vi "Calibrate Sensor.vi"(0 "Sensor":T4={"Sensor Name"="AI 0", "Sensor Info"={"Manufacturer"="", "Model"="", "Serial Number"=""}, "Last Cal Info"={"Last Calibration Date"=3153138208.25, "Calibrator"="", "Cal Duration"=0}, "Voltage Range"={"High Limit"=0.0, "Low Limit"=10.0}, "EGU Range"={"High Limit"=0.0, "Low Limit"=10.0}, "Units"="Volts", "Calibration Type"=enum."Calibrate Analog", "EGU List"=[0.0, 10000.0], "Voltage List"=[0.0, 5.0], "Coefficients"=[3.658184866139891e-14, 1999.9999999999998], "Order"=1, "Algorithm"=enum."SVD", "Max Error % of Full Scale"=0.0, "Max Mean Squared Error"=0.0, "Use Error %"=FALSE, "Use MSE"=FALSE, "Allow Manual Entry"=FALSE, "Max Stability Error"=2.0, "Max Error % of Reading"=0.0, "Use Error % of Reading"=FALSE}, 1 "System Ref":tag, 2 "TCP Stream Ref":refnum<vi>, 5 "Channel Info":T5={"Channel"="0-10V AI #0", "Description"="0-10V AI #0", "Acquire"=FALSE, "Sensor"="AI 0", "Chg Sensor"=FALSE, "Cal Date"="", "Offset"=0.0, "Span"=0.0, "Cal"=FALSE, "Test Limits"=FALSE, "Type"="", "Data Index"=0}, 7 "Cal Base Path":path, 9 "System Type":T1, 11 "Devices":T2=[{"Device"=2, "Channels"=[{"Channel ID"="OB0!SC1!MD2!0", "Channel Name"="0-10V AI #0 TRDC.1", "Channel Type"=enum."Voltage", "Selected Sensor"="WTI func gen", "Alarm Config"={"Action"=enum."Disabled", "Low Limit"=0.0, "High Limit"=0.0}, "Thermocouple Info"={"Thermocouple Type"=0, "Temperature Units"=0, "Temperature Low Limit"=0.0, "Temperature High Limit"=0.0, "CJC Sensor Type"=0, "Thermistor Excitation"=0, "CJC Channel ID"=0, "Dedicated CJTEMP for Channel"=0, "Use CALGND"=0, "Dedicated CALGND for Channel"=0}}, {"Channel ID"="OB0!SC1!MD1!0", "Channel Name"="J-TYPE TC #0", "Channel Type"=enum."Thermocouple", "Selected Sensor"="Hardware", "Alarm Config"={"Action"=enum."Disabled", "Low Limit"=0.0, "High Limit"=0.0}, "Thermocouple Info"={"Thermocouple Type"=2, "Temperature Units"=0, "Temperature Low Limit"=-60.0, "Temperature High Limit"=200.0, "CJC Sensor Type"=1, "Thermistor Excitation"=0, "CJC Channel ID"=0, "Dedicated CJTEMP for Channel"=0, "Use CALGND"=0, "Dedicated CALGND for Channel"=0}}, {"Channel ID"="OB0!SC1!MD1!1", "Channel Name"="J-TYPE TC #1", "Channel Type"=enum."Thermocouple", "Selected Sensor"="Hardware", "Alarm Config"={"Action"=enum."Disabled", "Low Limit"=0.0, "High Limit"=0.0}, "Thermocouple Info"={"Thermocouple Type"=2, "Temperature Units"=0, "Temperature Low Limit"=-60.0, "Temperature High Limit"=200.0, "CJC Sensor Type"=1, "Thermistor Excitation"=0, "CJC Channel ID"=0, "Dedicated CJTEMP for Channel"=0, "Use CALGND"=0, "Dedicated CALGND for Channel"=0}}, {"Channel ID"="OB0!SC1!MD1!2", "Channel Name"="J-TYPE TC #2", "Channel Type"=enum."Thermocouple", "Selected Sensor"="Hardware", "Alarm Config"={"Action"=enum."Disabled", "Low Limit"=0.0, "High Limit"=0.0}, "Thermocouple Info"={"Thermocouple Type"=2, "Temperature Units"=0, "Temperature Low Limit"=-60.0, "Temperature High Limit"=200.0, "CJC Sensor Type"=1, "Thermistor Excitation"=0, "CJC Channel ID"=0, "Dedicated CJTEMP for Channel"=0, "Use CALGND"=0, "Dedicated CALGND for Channel"=0}}, {"Channel ID"="OB0!SC1!MD1!3", "Channel Name"="J-TYPE TC #3", "Channel Type"=enum."Thermocouple", "Selected Sensor"="Hardware", "Alarm Config"={"Action"=enum."Disabled", "Low Limit"=0.0, "High Limit"=0.0}, "Thermocouple Info"={"Thermocouple Type"=2, "Temperature Units"=0, "Temperature Low Limit"=-60.0, "Temperature High Limit"=200.0, "CJC Sensor Type"=1, "Thermistor Excitation"=0, "CJC Channel ID"=0, "Dedicated CJTEMP for Channel"=0, "Use CALGND"=0, "Dedicated CALGND for Channel"=0}}, {"Channel ID"="OB0!SC1!MD1!4", "Channel Name"="J-TYPE TC #4", "Channel Type"=enum."Thermocouple", "Selected Sensor"="Hardware", "Alarm Config"={"Action"=enum."Disabled", "Low Limit"=0.0, "High Limit"=0.0}, "Thermocouple Info"={"Thermocouple Type"=2, "Temperature Units"=0, "Temperature Low Limit"=-60.0, "Temperature High Limit"=200.0, "CJC Sensor Type"=1, "Thermistor Excitation"=0, "CJC Channel ID"=0, "Dedicated CJTEMP for Channel"=0, "Use CALGND"=0, "Dedicated CALGND for Channel"=0}}, {"Channel ID"="OB0!SC1!MD1!5", "Channel Name"="J-TYPE TC #5", "Channel Type"=enum."Thermocouple", "Selected Sensor"="Hardware", "Alarm Config"={"Action"=enum."Disabled", "Low Limit"=0.0, "High Limit"=0.0}, "Thermocouple Info"={"Thermocouple Type"=2, "Temperature Units"=0, "Temperature Low Limit"=-60.0, "Temperature High Limit"=200.0, "CJC Sensor Type"=1, "Thermistor Excitation"=0, "CJC Channel ID"=0, "Dedicated CJTEMP for Channel"=0, "Use CALGND"=0, "Dedicated CALGND for Channel"=0}}, {"Channel ID"="OB0!SC1!MD1!6", "Channel Name"="J-TYPE TC #6", "Channel Type"=enum."Thermocouple", "Selected Sensor"="Hardware", "Alarm Config"={"Action"=enum."Disabled", "Low Limit"=0.0, "High Limit"=0.0}, "Thermocouple Info"={"Thermocouple Type"=2, "Temperature Units"=0, "Temperature Low Limit"=-60.0, "Temperature High Limit"=200.0, "CJC Sensor Type"=1, "Thermistor Excitation"=0, "CJC Channel ID"=0, "Dedicated CJTEMP for Channel"=0, "Use CALGND"=0, "Dedicated CALGND for Channel"=0}}, {"Channel ID"="OB0!SC1!MD1!7", "Channel Name"="J-TYPE TC #7", "Channel Type"=enum."Thermocouple", "Selected Sensor"="Hardware", "Alarm Config"={"Action"=enum."Disabled", "Low Limit"=0.0, "High Limit"=0.0}, "Thermocouple Info"={"Thermocouple Type"=2, "Temperature Units"=0, "Temperature Low Limit"=-60.0, "Temperature High Limit"=200.0, "CJC Sensor Type"=1, "Thermistor Excitation"=0, "CJC Channel ID"=0, "Dedicated CJTEMP for Channel"=0, "Use CALGND"=0, "Dedicated CALGND for Channel"=0}}, {"Channel ID"="OB0!SC1!MD1!8", "Channel Name"="J-TYPE TC #8", "Channel Type"=enum."Thermocouple", "Selected Sensor"="Hardware", "Alarm Config"={"Action"=enum."Disabled", "Low Limit"=0.0, "High Limit"=0.0}, "Thermocouple Info"={"Thermocouple Type"=2, "Temperature Units"=0, "Temperature Low Limit"=-60.0, "Temperature High Limit"=200.0, "CJC Sensor Type"=1, "Thermistor Excitation"=0, "CJC Channel ID"=0, "Dedicated CJTEMP for Channel"=0, "Use CALGND"=0, "Dedicated CALGND for Channel"=0}}, {"Channel ID"="OB0!SC1!MD1!9", "Channel Name"="J-TYPE TC #9", "Channel Type"=enum."Thermocouple", "Selected Sensor"="Hardware", "Alarm Config"={"Action"=enum."Disabled", "Low Limit"=0.0, "High Limit"=0.0}, "Thermocouple Info"={"Thermocouple Type"=2, "Temperature Units"=0, "Temperature Low Limit"=-60.0, "Temperature High Limit"=200.0, "CJC Sensor Type"=1, "Thermistor Excitation"=0, "CJC Channel ID"=0, "Dedicated CJTEMP for Channel"=0, "Use CALGND"=0, "Dedicated CALGND for Channel"=0}}, {"Channel ID"="OB0!SC1!MD1!10", "Channel Name"="J-TYPE TC #10", "Channel Type"=enum."Thermocouple", "Selected Sensor"="Hardware", "Alarm Config"={"Action"=enum."Disabled", "Low Limit"=0.0, "High Limit"=0.0}, "Thermocouple Info"={"Thermocouple Type"=2, "Temperature Units"=0, "Temperature Low Limit"=-60.0, "Temperature High Limit"=200.0, "CJC Sensor Type"=1, "Thermistor Excitation"=0, "CJC Channel ID"=0, "Dedicated CJTEMP for Channel"=0, "Use CALGND"=0, "Dedicated CALGND for Channel"=0}}, {"Channel ID"="OB0!SC1!MD1!11", "Channel Name"="J-TYPE TC #11", "Channel Type"=enum."Thermocouple", "Selected Sensor"="Hardware", "Alarm Config"={"Action"=enum."Disabled", "Low Limit"=0.0, "High Limit"=0.0}, "Thermocouple Info"={"Thermocouple Type"=2, "Temperature Units"=0, "Temperature Low Limit"=-60.0, "Temperature High Limit"=200.0, "CJC Sensor Type"=1, "Thermistor Excitation"=0, "CJC Channel ID"=0, "Dedicated CJTEMP for Channel"=0, "Use CALGND"=0, "Dedicated CALGND for Channel"=0}}, {"Channel ID"="OB0!SC1!MD1!12", "Channel Name"="J-TYPE TC #12", "Channel Type"=enum."Thermocouple", "Selected Sensor"="Hardware", "Alarm Config"={"Action"=enum."Disabled", "Low Limit"=0.0, "High Limit"=0.0}, "Thermocouple Info"={"Thermocouple Type"=2, "Temperature Units"=0, "Temperature Low Limit"=-60.0, "Temperature High Limit"=200.0, "CJC Sensor Type"=1, "Thermistor Excitation"=0, "CJC Channel ID"=0, "Dedicated CJTEMP for Channel"=0, "Use CALGND"=0, "Dedicated CALGND for Channel"=0}}, {"Channel ID"="OB0!SC1!MD1!13", "Channel Name"="J-TYPE TC #13", "Channel Type"=enum."Thermocouple", "Selected Sensor"="Hardware", "Alarm Config"={"Action"=enum."Disabled", "Low Limit"=0.0, "High Limit"=0.0}, "Thermocouple Info"={"Thermocouple Type"=2, "Temperature Units"=0, "Temperature Low Limit"=-60.0, "Temperature High Limit"=200.0, "CJC Sensor Type"=1, "Thermistor Excitation"=0, "CJC Channel ID"=0, "Dedicated CJTEMP for Channel"=0, "Use CALGND"=0, "Dedicated CALGND for Channel"=0}}, {"Channel ID"="OB0!SC1!MD1!14", "Channel Name"="J-TYPE TC #14", "Channel Type"=enum."Thermocouple", "Selected Sensor"="Hardware", "Alarm Config"={"Action"=enum."Disabled", "Low Limit"=0.0, "High Limit"=0.0}, "Thermocouple Info"={"Thermocouple Type"=2, "Temperature Units"=0, "Temperature Low Limit"=-60.0, "Temperature High Limit"=200.0, "CJC Sensor Type"=1, "Thermistor Excitation"=0, "CJC Channel ID"=0, "Dedicated CJTEMP for Channel"=0, "Use CALGND"=0, "Dedicated CALGND for Channel"=0}}, {"Channel ID"="OB0!SC1!MD1!15", "Channel Name"="J-TYPE TC #15", "Channel Type"=enum."Thermocouple", "Selected Sensor"="Hardware", "Alarm Config"={"Action"=enum."Disabled", "Low Limit"=0.0, "High Limit"=0.0}, "Thermocouple Info"={"Thermocouple Type"=2, "Temperature Units"=0, "Temperature Low Limit"=-60.0, "Temperature High Limit"=200.0, "CJC Sensor Type"=1, "Thermistor Excitation"=0, "CJC Channel ID"=0, "Dedicated CJTEMP for Channel"=0, "Use CALGND"=0, "Dedicated CALGND for Channel"=0}}, {"Channel ID"="OB0!SC1!MD1!16", "Channel Name"="T-TYPE TC #16", "Channel Type"=enum."Thermocouple", "Selected Sensor"="Hardware", "Alarm Config"={"Action"=enum."Disabled", "Low Limit"=0.0, "High Limit"=0.0}, "Thermocouple Info"={"Thermocouple Type"=6, "Temperature Units"=0, "Temperature Low Limit"=-60.0, "Temperature High Limit"=200.0, "CJC Sensor Type"=1, "Thermistor Excitation"=0, "CJC Channel ID"=0, "Dedicated CJTEMP for Channel"=0, "Use CALGND"=0, "Dedicated CALGND for Channel"=0}}, {"Channel ID"="OB0!SC1!MD1!17", "Channel Name"="T-TYPE TC #17", "Channel Type"=enum."Thermocouple", "Selected Sensor"="Hardware", "Alarm Config"={"Action"=enum."Disabled", "Low Limit"=0.0, "High Limit"=0.0}, "Thermocouple Info"={"Thermocouple Type"=6, "Temperature Units"=0, "Temperature Low Limit"=-60.0, "Temperature High Limit"=200.0, "CJC Sensor Type"=1, "Thermistor Excitation"=0, "CJC Channel ID"=0, "Dedicated CJTEMP for Channel"=0, "Use CALGND"=0, "Dedicated CALGND for Channel"=0}}, {"Channel ID"="OB0!SC1!MD1!18", "Channel Name"="T-TYPE TC #18", "Channel Type"=enum."Thermocouple", "Selected Sensor"="Hardware", "Alarm Config"={"Action"=enum."Disabled", "Low Limit"=0.0, "High Limit"=0.0}, "Thermocouple Info"={"Thermocouple Type"=6, "Temperature Units"=0, "Temperature Low Limit"=-60.0, "Temperature High Limit"=200.0, "CJC Sensor Type"=1, "Thermistor Excitation"=0, "CJC Channel ID"=0, "Dedicated CJTEMP for Channel"=0, "Use CALGND"=0, "Dedicated CALGND for Channel"=0}}, {"Channel ID"="OB0!SC1!MD1!19", "Channel Name"="T-TYPE TC #19", "Channel Type"=enum."Thermocouple", "Selected Sensor"="Hardware", "Alarm Config"={"Action"=enum."Disabled", "Low Limit"=0.0, "High Limit"=0.0}, "Thermocouple Info"={"Thermocouple Type"=6, "Temperature Units"=0, "Temperature Low Limit"=-60.0, "Temperature High Limit"=200.0, "CJC Sensor Type"=1, "Thermistor Excitation"=0, "CJC Channel ID"=0, "Dedicated CJTEMP for Channel"=0, "Use CALGND"=0, "Dedicated CALGND for Channel"=0}}, {"Channel ID"="OB0!SC1!MD1!20", "Channel Name"="T-TYPE TC #20", "Channel Type"=enum."Thermocouple", "Selected Sensor"="Hardware", "Alarm Config"={"Action"=enum."Disabled", "Low Limit"=0.0, "High Limit"=0.0}, "Thermocouple Info"={"Thermocouple Type"=6, "Temperature Units"=0, "Temperature Low Limit"=-60.0, "Temperature High Limit"=200.0, "CJC Sensor Type"=1, "Thermistor Excitation"=0, "CJC Channel ID"=0, "Dedicated CJTEMP for Channel"=0, "Use CALGND"=0, "Dedicated CALGND for Channel"=0}}, {"Channel ID"="OB0!SC1!MD1!21", "Channel Name"="T-TYPE TC #21", "Channel Type"=enum."Thermocouple", "Selected Sensor"="Hardware", "Alarm Config"={"Action"=enum."Disabled", "Low Limit"=0.0, "High Limit"=0.0}, "Thermocouple Info"={"Thermocouple Type"=6, "Temperature Units"=0, "Temperature Low Limit"=-60.0, "Temperature High Limit"=200.0, "CJC Sensor Type"=1, "Thermistor Excitation"=0, "CJC Channel ID"=0, "Dedicated CJTEMP for Channel"=0, "Use CALGND"=0, "Dedicated CALGND for Channel"=0}}, {"Channel ID"="OB0!SC1!MD1!22", "Channel Name"="T-TYPE TC #22", "Channel Type"=enum."Thermocouple", "Selected Sensor"="Hardware", "Alarm Config"={"Action"=enum."Disabled", "Low Limit"=0.0, "High Limit"=0.0}, "Thermocouple Info"={"Thermocouple Type"=6, "Temperature Units"=0, "Temperature Low Limit"=-60.0, "Temperature High Limit"=200.0, "CJC Sensor Type"=1, "Thermistor Excitation"=0, "CJC Channel ID"=0, "Dedicated CJTEMP for Channel"=0, "Use CALGND"=0, "Dedicated CALGND for Channel"=0}}, {"Channel ID"="OB0!SC1!MD1!23", "Channel Name"="T-TYPE TC #23", "Channel Type"=enum."Thermocouple", "Selected Sensor"="Hardware", "Alarm Config"={"Action"=enum."Disabled", "Low Limit"=0.0, "High Limit"=0.0}, "Thermocouple Info"={"Thermocouple Type"=6, "Temperature Units"=0, "Temperature Low Limit"=-60.0, "Temperature High Limit"=200.0, "CJC Sensor Type"=1, "Thermistor Excitation"=0, "CJC Channel ID"=0, "Dedicated CJTEMP for Channel"=0, "Use CALGND"=0, "Dedicated CALGND for Channel"=0}}, {"Channel ID"="OB0!SC1!MD1!24", "Channel Name"="T-TYPE TC #24", "Channel Type"=enum."Thermocouple", "Selected Sensor"="Hardware", "Alarm Config"={"Action"=enum."Disabled", "Low Limit"=0.0, "High Limit"=0.0}, "Thermocouple Info"={"Thermocouple Type"=6, "Temperature Units"=0, "Temperature Low Limit"=-60.0, "Temperature High Limit"=200.0, "CJC Sensor Type"=1, "Thermistor Excitation"=0, "CJC Channel ID"=0, "Dedicated CJTEMP for Channel"=0, "Use CALGND"=0, "Dedicated CALGND for Channel"=0}}, {"Channel ID"="OB0!SC1!MD1!25", "Channel Name"="T-TYPE TC #25", "Channel Type"=enum."Thermocouple", "Selected Sensor"="Hardware", "Alarm Config"={"Action"=enum."Disabled", "Low Limit"=0.0, "High Limit"=0.0}, "Thermocouple Info"={"Thermocouple Type"=6, "Temperature Units"=0, "Temperature Low Limit"=-60.0, "Temperature High Limit"=200.0, "CJC Sensor Type"=1, "Thermistor Excitation"=0, "CJC Channel ID"=0, "Dedicated CJTEMP for Channel"=0, "Use CALGND"=0, "Dedicated CALGND for Channel"=0}}, {"Channel ID"="OB0!SC1!MD1!26", "Channel Name"="T-TYPE TC #26", "Channel Type"=enum."Thermocouple", "Selected Sensor"="Hardware", "Alarm Config"={"Action"=enum."Disabled", "Low Limit"=0.0, "High Limit"=0.0}, "Thermocouple Info"={"Thermocouple Type"=6, "Temperature Units"=0, "Temperature Low Limit"=-60.0, "Temperature High Limit"=200.0, "CJC Sensor Type"=1, "Thermistor Excitation"=0, "CJC Channel ID"=0, "Dedicated CJTEMP for Channel"=0, "Use CALGND"=0, "Dedicated CALGND for Channel"=0}}, {"Channel ID"="OB0!SC1!MD1!27", "Channel Name"="T-TYPE TC #27", "Channel Type"=enum."Thermocouple", "Selected Sensor"="Hardware", "Alarm Config"={"Action"=enum."Disabled", "Low Limit"=0.0, "High Limit"=0.0}, "Thermocouple Info"={"Thermocouple Type"=6, "Temperature Units"=0, "Temperature Low Limit"=-60.0, "Temperature High Limit"=200.0, "CJC Sensor Type"=1, "Thermistor Excitation"=0, "CJC Channel ID"=0, "Dedicated CJTEMP for Channel"=0, "Use CALGND"=0, "Dedicated CALGND for Channel"=0}}, {"Channel ID"="OB0!SC1!MD1!28", "Channel Name"="T-TYPE TC #28", "Channel Type"=enum."Thermocouple", "Selected Sensor"="Hardware", "Alarm Config"={"Action"=enum."Disabled", "Low Limit"=0.0, "High Limit"=0.0}, "Thermocouple Info"={"Thermocouple Type"=6, "Temperature Units"=0, "Temperature Low Limit"=-60.0, "Temperature High Limit"=200.0, "CJC Sensor Type"=1, "Thermistor Excitation"=0, "CJC Channel ID"=0, "Dedicated CJTEMP for Channel"=0, "Use CALGND"=0, "Dedicated CALGND for Channel"=0}}, {"Channel ID"="OB0!SC1!MD1!29", "Channel Name"="T-TYPE TC #29", "Channel Type"=enum."Thermocouple", "Selected Sensor"="Hardware", "Alarm Config"={"Action"=enum."Disabled", "Low Limit"=0.0, "High Limit"=0.0}, "Thermocouple Info"={"Thermocouple Type"=6, "Temperature Units"=0, "Temperature Low Limit"=-60.0, "Temperature High Limit"=200.0, "CJC Sensor Type"=1, "Thermistor Excitation"=0, "CJC Channel ID"=0, "Dedicated CJTEMP for Channel"=0, "Use CALGND"=0, "Dedicated CALGND for Channel"=0}}, {"Channel ID"="OB0!SC1!MD1!30", "Channel Name"="T-TYPE TC #30", "Channel Type"=enum."Thermocouple", "Selected Sensor"="Hardware", "Alarm Config"={"Action"=enum."Disabled", "Low Limit"=0.0, "High Limit"=0.0}, "Thermocouple Info"={"Thermocouple Type"=6, "Temperature Units"=0, "Temperature Low Limit"=-60.0, "Temperature High Limit"=200.0, "CJC Sensor Type"=1, "Thermistor Excitation"=0, "CJC Channel ID"=0, "Dedicated CJTEMP for Channel"=0, "Use CALGND"=0, "Dedicated CALGND for Channel"=0}}, {"Channel ID"="OB0!SC1!MD1!31", "Channel Name"="T-TYPE TC #31", "Channel Type"=enum."Thermocouple", "Selected Sensor"="Hardware", "Alarm Config"={"Action"=enum."Disabled", "Low Limit"=0.0, "High Limit"=0.0}, "Thermocouple Info"={"Thermocouple Type"=6, "Temperature Units"=0, "Temperature Low Limit"=-60.0, "Temperature High Limit"=200.0, "CJC Sensor Type"=1, "Thermistor Excitation"=0, "CJC Channel ID"=0, "Dedicated CJTEMP for Channel"=0, "Use CALGND"=0, "Dedicated CALGND for Channel"=0}}, {"Channel ID"="OB0!SC1!MD2!0", "Channel Name"="0-10V AI #0 TRDC.1", "Channel Type"=enum."Voltage", "Selected Sensor"="WTI func gen", "Alarm Config"={"Action"=enum."Disabled", "Low Limit"=0.0, "High Limit"=0.0}, "Thermocouple Info"={"Thermocouple Type"=0, "Temperature Units"=0, "Temperature Low Limit"=-60.0, "Temperature High Limit"=200.0, "CJC Sensor Type"=1, "Thermistor Excitation"=0, "CJC Channel ID"=0, "Dedicated CJTEMP for Channel"=0, "Use CALGND"=0, "Dedicated CALGND for Channel"=0}}, {"Channel ID"="OB0!SC1!MD2!1", "Channel Name"="0-10V AI #1 TRDC.2", "Channel Type"=enum."Voltage", "Selected Sensor"="WTI func gen", "Alarm Config"={"Action"=enum."Disabled", "Low Limit"=0.0, "High Limit"=0.0}, "Thermocouple Info"={"Thermocouple Type"=0, "Temperature Units"=0, "Temperature Low Limit"=-60.0, "Temperature High Limit"=200.0, "CJC Sensor Type"=1, "Thermistor Excitation"=0, "CJC Channel ID"=0, "Dedicated CJTEMP for Channel"=0, "Use CALGND"=0, "Dedicated CALGND for Channel"=0}}, {"Channel ID"="OB0!SC1!MD2!2", "Channel Name"="0-10V AI #2 TRDC.3", "Channel Type"=enum."Voltage", "Selected Sensor"="WTI func gen", "Alarm Config"={"Action"=enum."Disabled", "Low Limit"=0.0, "High Limit"=0.0}, "Thermocouple Info"={"Thermocouple Type"=0, "Temperature Units"=0, "Temperature Low Limit"=-60.0, "Temperature High Limit"=200.0, "CJC Sensor Type"=1, "Thermistor Excitation"=0, "CJC Channel ID"=0, "Dedicated CJTEMP for Channel"=0, "Use CALGND"=0, "Dedicated CALGND for Channel"=0}}, {"Channel ID"="OB0!SC1!MD2!3", "Channel Name"="0-10V AI #3 TRDC.4", "Channel Type"=enum."Voltage", "Selected Sensor"="WTI func gen", "Alarm Config"={"Action"=enum."Disabled", "Low Limit"=0.0, "High Limit"=0.0}, "Thermocouple Info"={"Thermocouple Type"=0, "Temperature Units"=0, "Temperature Low Limit"=-60.0, "Temperature High Limit"=200.0, "CJC Sensor Type"=1, "Thermistor Excitation"=0, "CJC Channel ID"=0, "Dedicated CJTEMP for Channel"=0, "Use CALGND"=0, "Dedicated CALGND for Channel"=0}}, {"Channel ID"="OB0!SC1!MD2!4", "Channel Name"="0-10V AI #4 TRDC.5", "Channel Type"=enum."Voltage", "Selected Sensor"="WTI func gen", "Alarm Config"={"Action"=enum."Disabled", "Low Limit"=0.0, "High Limit"=0.0}, "Thermocouple Info"={"Thermocouple Type"=0, "Temperature Units"=0, "Temperature Low Limit"=-60.0, "Temperature High Limit"=200.0, "CJC Sensor Type"=1, "Thermistor Excitation"=0, "CJC Channel ID"=0, "Dedicated CJTEMP for Channel"=0, "Use CALGND"=0, "Dedicated CALGND for Channel"=0}}, {"Channel ID"="OB0!SC1!MD2!5", "Channel Name"="0-10V AI #5 TRDC.6", "Channel Type"=enum."Voltage", "Selected Sensor"="WTI func gen", "Alarm Config"={"Action"=enum."Disabled", "Low Limit"=0.0, "High Limit"=0.0}, "Thermocouple Info"={"Thermocouple Type"=0, "Temperature Units"=0, "Temperature Low Limit"=-60.0, "Temperature High Limit"=200.0, "CJC Sensor Type"=1, "Thermistor Excitation"=0, "CJC Channel ID"=0, "Dedicated CJTEMP for Channel"=0, "Use CALGND"=0, "Dedicated CALGND for Channel"=0}}, {"Channel ID"="OB0!SC1!MD2!6", "Channel Name"="0-10V AI #6 TRDC.7", "Channel Type"=enum."Voltage", "Selected Sensor"="WTI func gen", "Alarm Config"={"Action"=enum."Disabled", "Low Limit"=0.0, "High Limit"=0.0}, "Thermocouple Info"={"Thermocouple Type"=0, "Temperature Units"=0, "Temperature Low Limit"=-60.0, "Temperature High Limit"=200.0, "CJC Sensor Type"=1, "Thermistor Excitation"=0, "CJC Channel ID"=0, "Dedicated CJTEMP for Channel"=0, "Use CALGND"=0, "Dedicated CALGND for Channel"=0}}, {"Channel ID"="OB0!SC1!MD2!7", "Channel Name"="0-10V AI #7 TRDC.8", "Channel Type"=enum."Voltage", "Selected Sensor"="WTI func gen", "Alarm Config"={"Action"=enum."Disabled", "Low Limit"=0.0, "High Limit"=0.0}, "Thermocouple Info"={"Thermocouple Type"=0, "Temperature Units"=0, "Temperature Low Limit"=-60.0, "Temperature High Limit"=200.0, "CJC Sensor Type"=1, "Thermistor Excitation"=0, "CJC Channel ID"=0, "Dedicated CJTEMP for Channel"=0, "Use CALGND"=0, "Dedicated CALGND for Channel"=0}}, {"Channel ID"="OB0!SC1!MD2!8", "Channel Name"="0-10V AI #8 TRDC.9", "Channel Type"=enum."Voltage", "Selected Sensor"="WTI func gen", "Alarm Config"={"Action"=enum."Disabled", "Low Limit"=0.0, "High Limit"=0.0}, "Thermocouple Info"={"Thermocouple Type"=0, "Temperature Units"=0, "Temperature Low Limit"=-60.0, "Temperature High Limit"=200.0, "CJC Sensor Type"=1, "Thermistor Excitation"=0, "CJC Channel ID"=0, "Dedicated CJTEMP for Channel"=0, "Use CALGND"=0, "Dedicated CALGND for Channel"=0}}, {"Channel ID"="OB0!SC1!MD2!9", "Channel Name"="0-10V AI #9 TRDC.10", "Channel Type"=enum."Voltage", "Selected Sensor"="WTI func gen", "Alarm Config"={"Action"=enum."Disabled", "Low Limit"=0.0, "High Limit"=0.0}, "Thermocouple Info"={"Thermocouple Type"=0, "Temperature Units"=0, "Temperature Low Limit"=-60.0, "Temperature High Limit"=200.0, "CJC Sensor Type"=1, "Thermistor Excitation"=0, "CJC Channel ID"=0, "Dedicated CJTEMP for Channel"=0, "Use CALGND"=0, "Dedicated CALGND for Channel"=0}}, {"Channel ID"="OB0!SC1!MD2!10", "Channel Name"="0-10V AI #10 TRDC.11", "Channel Type"=enum."Voltage", "Selected Sensor"="WTI func gen", "Alarm Config"={"Action"=enum."Disabled", "Low Limit"=0.0, "High Limit"=0.0}, "Thermocouple Info"={"Thermocouple Type"=0, "Temperature Units"=0, "Temperature Low Limit"=-60.0, "Temperature High Limit"=200.0, "CJC Sensor Type"=1, "Thermistor Excitation"=0, "CJC Channel ID"=0, "Dedicated CJTEMP for Channel"=0, "Use CALGND"=0, "Dedicated CALGND for Channel"=0}}, {"Channel ID"="OB0!SC1!MD2!11", "Channel Name"="0-10V AI #11 TRDC.12", "Channel Type"=enum."Voltage", "Selected Sensor"="WTI func gen", "Alarm Config"={"Action"=enum."Disabled", "Low Limit"=0.0, "High Limit"=0.0}, "Thermocouple Info"={"Thermocouple Type"=0, "Temperature Units"=0, "Temperature Low Limit"=-60.0, "Temperature High Limit"=200.0, "CJC Sensor Type"=1, "Thermistor Excitation"=0, "CJC Channel ID"=0, "Dedicated CJTEMP for Channel"=0, "Use CALGND"=0, "Dedicated CALGND for Channel"=0}}, {"Channel ID"="OB0!SC1!MD2!12", "Channel Name"="0-10V AI #12 TRDC.13", "Channel Type"=enum."Voltage", "Selected Sensor"="WTI func gen", "Alarm Config"={"Action"=enum."Disabled", "Low Limit"=0.0, "High Limit"=0.0}, "Thermocouple Info"={"Thermocouple Type"=0, "Temperature Units"=0, "Temperature Low Limit"=-60.0, "Temperature High Limit"=200.0, "CJC Sensor Type"=1, "Thermistor Excitation"=0, "CJC Channel ID"=0, "Dedicated CJTEMP for Channel"=0, "Use CALGND"=0, "Dedicated CALGND for Channel"=0}}, {"Channel ID"="OB0!SC1!MD2!13", "Channel Name"="0-10V AI #13 TRDC.14", "Channel Type"=enum."Voltage", "Selected Sensor"="WTI func gen", "Alarm Config"={"Action"=enum."Disabled", "Low Limit"=0.0, "High Limit"=0.0}, "Thermocouple Info"={"Thermocouple Type"=0, "Temperature Units"=0, "Temperature Low Limit"=-60.0, "Temperature High Limit"=200.0, "CJC Sensor Type"=1, "Thermistor Excitation"=0, "CJC Channel ID"=0, "Dedicated CJTEMP for Channel"=0, "Use CALGND"=0, "Dedicated CALGND for Channel"=0}}, {"Channel ID"="OB0!SC1!MD2!14", "Channel Name"="0-10V AI #14 TRDC.15", "Channel Type"=enum."Voltage", "Selected Sensor"="WTI func gen", "Alarm Config"={"Action"=enum."Disabled", "Low Limit"=0.0, "High Limit"=0.0}, "Thermocouple Info"={"Thermocouple Type"=0, "Temperature Units"=0, "Temperature Low Limit"=-60.0, "Temperature High Limit"=200.0, "CJC Sensor Type"=1, "Thermistor Excitation"=0, "CJC Channel ID"=0, "Dedicated CJTEMP for Channel"=0, "Use CALGND"=0, "Dedicated CALGND for Channel"=0}}, {"Channel ID"="OB0!SC1!MD2!15", "Channel Name"="0-10V AI #15 TRDC.16", "Channel Type"=enum."Voltage", "Selected Sensor"="WTI func gen", "Alarm Config"={"Action"=enum."Disabled", "Low Limit"=0.0, "High Limit"=0.0}, "Thermocouple Info"={"Thermocouple Type"=0, "Temperature Units"=0, "Temperature Low Limit"=-60.0, "Temperature High Limit"=200.0, "CJC Sensor Type"=1, "Thermistor Excitation"=0, "CJC Channel ID"=0, "Dedicated CJTEMP for Channel"=0, "Use CALGND"=0, "Dedicated CALGND for Channel"=0}}]}] {"Channels"."Thermocouple Info"."Dedicated CALGND for Channel" items=["No", "Yes"]; "Channels"."Thermocouple Info"."Use CALGND" items=["No", "Yes"]; "Channels"."Thermocouple Info"."Dedicated CJTEMP for Channel" items=["No", "Yes"]; "Channels"."Thermocouple Info"."CJC Channel ID" items=["CJTEMP", "MTEMP"]; "Channels"."Thermocouple Info"."Thermistor Excitation" items=["Voltage Reference", "Current Reference"]; "Channels"."Thermocouple Info"."CJC Sensor Type" items=["IC Sensor", "Thermistor"]; "Channels"."Thermocouple Info"."Temperature Units" items=["Celsius", "Fahrenheit", "Kelvin", "Rankine"]; "Channels"."Thermocouple Info"."Temperature Low Limit" format="%0.3f"; "Channels"."Thermocouple Info"."Temperature High Limit" format="%0.3f"; "Channels"."Thermocouple Info"."Thermocouple Type" items=["B Thermocouple", "E Thermocouple", "J Thermocouple", "K Thermocouple", "R Thermocouple", "S Thermocouple", "T Thermocouple", "N Thermocouple"]; "Channels"."Alarm Config"."High Limit" format="%.2f"; "Channels"."Alarm Config"."Low Limit" format="%.2f"}, 12 "Sensors Info":T3(array[cluster])=[{"Sensor Name"="AI 0", "Sensor Info"={"Manufacturer"="", "Model"="", "Serial Number"=""}, "Last Cal Info"={"Last Calibration Date"=3154600440.828, "Calibrator"="", "Cal Duration"=0}, "Voltage Range"={"High Limit"=10.0, "Low Limit"=0.0}, "EGU Range"={"High Limit"=10.0, "Low Limit"=0.0}, "Units"="Volts", "Calibration Type"=enum."Calibrate Analog", "EGU List"=[0.0, 10.0], "Voltage List"=[0.0, 10.0], "Coefficients"=[-0.0, 1.0], "Order"=1, "Algorithm"=enum."SVD", "Max Error % of Full Scale"=0.0, "Max Mean Squared Error"=0.0, "Use Error %"=FALSE, "Use MSE"=FALSE, "Allow Manual Entry"=FALSE, "Max Stability Error"=2.0, "Max Error % of Reading"=0.0, "Use Error % of Reading"=FALSE}, {"Sensor Name"="AI 1", "Sensor Info"={"Manufacturer"="", "Model"="", "Serial Number"=""}, "Last Cal Info"={"Last Calibration Date"=3154600454.0, "Calibrator"="", "Cal Duration"=0}, "Voltage Range"={"High Limit"=10.0, "Low Limit"=0.0}, "EGU Range"={"High Limit"=10.0, "Low Limit"=0.0}, "Units"="Volts", "Calibration Type"=enum."Calibrate Analog", "EGU List"=[0.0, 10.0], "Voltage List"=[0.0, 10.0], "Coefficients"=[-0.0, 1.0], "Order"=1, "Algorithm"=enum."SVD", "Max Error % of Full Scale"=0.0, "Max Mean Squared Error"=0.0, "Use Error %"=FALSE, "Use MSE"=FALSE, "Allow Manual Entry"=FALSE, "Max Stability Error"=2.0, "Max Error % of Reading"=0.0, "Use Error % of Reading"=FALSE}, {"Sensor Name"="AI 10", "Sensor Info"={"Manufacturer"="", "Model"="", "Serial Number"=""}, "Last Cal Info"={"Last Calibration Date"=3154600527.828, "Calibrator"="", "Cal Duration"=0}, "Voltage Range"={"High Limit"=10.0, "Low Limit"=0.0}, "EGU Range"={"High Limit"=10.0, "Low Limit"=0.0}, "Units"="Volts", "Calibration Type"=enum."Calibrate Analog", "EGU List"=[0.0, 10.0], "Voltage List"=[0.0, 10.0], "Coefficients"=[2.656295322589486e-18, 0.9999999999999999], "Order"=1, "Algorithm"=enum."SVD", "Max Error % of Full Scale"=0.0, "Max Mean Squared Error"=0.0, "Use Error %"=FALSE, "Use MSE"=FALSE, "Allow Manual Entry"=FALSE, "Max Stability Error"=2.0, "Max Error % of Reading"=0.0, "Use Error % of Reading"=FALSE}, {"Sensor Name"="AI 11", "Sensor Info"={"Manufacturer"="", "Model"="", "Serial Number"=""}, "Last Cal Info"={"Last Calibration Date"=3154600533.671, "Calibrator"="", "Cal Duration"=0}, "Voltage Range"={"High Limit"=10.0, "Low Limit"=0.0}, "EGU Range"={"High Limit"=10.0, "Low Limit"=0.0}, "Units"="Volts", "Calibration Type"=enum."Calibrate Analog", "EGU List"=[0.0, 10.0], "Voltage List"=[0.0, 10.0], "Coefficients"=[-0.0, 1.0], "Order"=1, "Algorithm"=enum."SVD", "Max Error % of Full Scale"=0.0, "Max Mean Squared Error"=0.0, "Use Error %"=FALSE, "Use MSE"=FALSE, "Allow Manual Entry"=FALSE, "Max Stability Error"=2.0, "Max Error % of Reading"=0.0, "Use Error % of Reading"=FALSE}, {"Sensor Name"="AI 12", "Sensor Info"={"Manufacturer"="", "Model"="", "Serial Number"=""}, "Last Cal Info"={"Last Calibration Date"=3154600543.328, "Calibrator"="", "Cal Duration"=0}, "Voltage Range"={"High Limit"=10.0, "Low Limit"=0.0}, "EGU Range"={"High Limit"=10.0, "Low Limit"=0.0}, "Units"="Volts", "Calibration Type"=enum."Calibrate Analog", "EGU List"=[0.0, 10.0], "Voltage List"=[0.0, 10.0], "Coefficients"=[2.656295322589486e-18, 0.9999999999999999], "Order"=1, "Algorithm"=enum."SVD", "Max Error % of Full Scale"=0.0, "Max Mean Squared Error"=0.0, "Use Error %"=FALSE, "Use MSE"=FALSE, "Allow Manual Entry"=FALSE, "Max Stability Error"=2.0, "Max Error % of Reading"=0.0, "Use Error % of Reading"=FALSE}, {"Sensor Name"="AI 13", "Sensor Info"={"Manufacturer"="", "Model"="", "Serial Number"=""}, "Last Cal Info"={"Last Calibration Date"=3154600557.75, "Calibrator"="", "Cal Duration"=0}, "Voltage Range"={"High Limit"=10.0, "Low Limit"=0.0}, "EGU Range"={"High Limit"=10.0, "Low Limit"=0.0}, "Units"="Volts", "Calibration Type"=enum."Calibrate Analog", "EGU List"=[0.0, 10.0], "Voltage List"=[0.0, 10.0], "Coefficients"=[2.656295322589486e-18, 0.9999999999999999], "Order"=1, "Algorithm"=enum."SVD", "Max Error % of Full Scale"=0.0, "Max Mean Squared Error"=0.0, "Use Error %"=FALSE, "Use MSE"=FALSE, "Allow Manual Entry"=FALSE, "Max Stability Error"=2.0, "Max Error % of Reading"=0.0, "Use Error % of Reading"=FALSE}, {"Sensor Name"="AI 14", "Sensor Info"={"Manufacturer"="", "Model"="", "Serial Number"=""}, "Last Cal Info"={"Last Calibration Date"=3154600583.64, "Calibrator"="", "Cal Duration"=0}, "Voltage Range"={"High Limit"=10.0, "Low Limit"=0.0}, "EGU Range"={"High Limit"=10.0, "Low Limit"=0.0}, "Units"="Volts", "Calibration Type"=enum."Calibrate Analog", "EGU List"=[0.0, 10.0], "Voltage List"=[0.0, 10.0], "Coefficients"=[2.656295322589486e-18, 0.9999999999999999], "Order"=1, "Algorithm"=enum."SVD", "Max Error % of Full Scale"=0.0, "Max Mean Squared Error"=0.0, "Use Error %"=FALSE, "Use MSE"=FALSE, "Allow Manual Entry"=FALSE, "Max Stability Error"=2.0, "Max Error % of Reading"=0.0, "Use Error % of Reading"=FALSE}, {"Sensor Name"="AI 15", "Sensor Info"={"Manufacturer"="", "Model"="", "Serial Number"=""}, "Last Cal Info"={"Last Calibration Date"=3154600589.9839997, "Calibrator"="", "Cal Duration"=0}, "Voltage Range"={"High Limit"=10.0, "Low Limit"=0.0}, "EGU Range"={"High Limit"=10.0, "Low Limit"=0.0}, "Units"="Volts", "Calibration Type"=enum."Calibrate Analog", "EGU List"=[0.0, 10.0], "Voltage List"=[0.0, 10.0], "Coefficients"=[2.656295322589486e-18, 0.9999999999999999], "Order"=1, "Algorithm"=enum."SVD", "Max Error % of Full Scale"=0.0, "Max Mean Squared Error"=0.0, "Use Error %"=FALSE, "Use MSE"=FALSE, "Allow Manual Entry"=FALSE, "Max Stability Error"=2.0, "Max Error % of Reading"=0.0, "Use Error % of Reading"=FALSE}, {"Sensor Name"="AI 2", "Sensor Info"={"Manufacturer"="", "Model"="", "Serial Number"=""}, "Last Cal Info"={"Last Calibration Date"=3154600472.437, "Calibrator"="", "Cal Duration"=0}, "Voltage Range"={"High Limit"=10.0, "Low Limit"=0.0}, "EGU Range"={"High Limit"=10.0, "Low Limit"=0.0}, "Units"="Volts", "Calibration Type"=enum."Calibrate Analog", "EGU List"=[0.0, 10.0], "Voltage List"=[0.0, 10.0], "Coefficients"=[2.656295322589486e-18, 0.9999999999999999], "Order"=1, "Algorithm"=enum."SVD", "Max Error % of Full Scale"=0.0, "Max Mean Squared Error"=0.0, "Use Error %"=FALSE, "Use MSE"=FALSE, "Allow Manual Entry"=FALSE, "Max Stability Error"=2.0, "Max Error % of Reading"=0.0, "Use Error % of Reading"=FALSE}, {"Sensor Name"="AI 3", "Sensor Info"={"Manufacturer"="", "Model"="", "Serial Number"=""}, "Last Cal Info"={"Last Calibration Date"=3154600477.078, "Calibrator"="", "Cal Duration"=0}, "Voltage Range"={"High Limit"=10.0, "Low Limit"=0.0}, "EGU Range"={"High Limit"=10.0, "Low Limit"=0.0}, "Units"="Volts", "Calibration Type"=enum."Calibrate Analog", "EGU List"=[0.0, 10.0], "Voltage List"=[0.0, 10.0], "Coefficients"=[2.656295322589486e-18, 0.9999999999999999], "Order"=1, "Algorithm"=enum."SVD", "Max Error % of Full Scale"=0.0, "Max Mean Squared Error"=0.0, "Use Error %"=FALSE, "Use MSE"=FALSE, "Allow Manual Entry"=FALSE, "Max Stability Error"=2.0, "Max Error % of Reading"=0.0, "Use Error % of Reading"=FALSE}, {"Sensor Name"="AI 4", "Sensor Info"={"Manufacturer"="", "Model"="", "Serial Number"=""}, "Last Cal Info"={"Last Calibration Date"=3154600483.2339997, "Calibrator"="", "Cal Duration"=0}, "Voltage Range"={"High Limit"=10.0, "Low Limit"=0.0}, "EGU Range"={"High Limit"=10.0, "Low Limit"=0.0}, "Units"="Volts", "Calibration Type"=enum."Calibrate Analog", "EGU List"=[0.0, 10.0], "Voltage List"=[0.0, 10.0], "Coefficients"=[2.656295322589486e-18, 0.9999999999999999], "Order"=1, "Algorithm"=enum."SVD", "Max Error % of Full Scale"=0.0, "Max Mean Squared Error"=0.0, "Use Error %"=FALSE, "Use MSE"=FALSE, "Allow Manual Entry"=FALSE, "Max Stability Error"=2.0, "Max Error % of Reading"=0.0, "Use Error % of Reading"=FALSE}, {"Sensor Name"="AI 5", "Sensor Info"={"Manufacturer"="", "Model"="", "Serial Number"=""}, "Last Cal Info"={"Last Calibration Date"=3154600489.578, "Calibrator"="", "Cal Duration"=0}, "Voltage Range"={"High Limit"=10.0, "Low Limit"=0.0}, "EGU Range"={"High Limit"=10.0, "Low Limit"=0.0}, "Units"="Volts", "Calibration Type"=enum."Calibrate Analog", "EGU List"=[0.0, 10.0], "Voltage List"=[0.0, 10.0], "Coefficients"=[2.656295322589486e-18, 0.9999999999999999], "Order"=1, "Algorithm"=enum."SVD", "Max Error % of Full Scale"=0.0, "Max Mean Squared Error"=0.0, "Use Error %"=FALSE, "Use MSE"=FALSE, "Allow Manual Entry"=FALSE, "Max Stability Error"=2.0, "Max Error % of Reading"=0.0, "Use Error % of Reading"=FALSE}, {"Sensor Name"="AI 6", "Sensor Info"={"Manufacturer"="", "Model"="", "Serial Number"=""}, "Last Cal Info"={"Last Calibration Date"=3154600496.0309997, "Calibrator"="", "Cal Duration"=0}, "Voltage Range"={"High Limit"=10.0, "Low Limit"=0.0}, "EGU Range"={"High Limit"=10.0, "Low Limit"=0.0}, "Units"="Volts", "Calibration Type"=enum."Calibrate Analog", "EGU List"=[0.0, 10.0], "Voltage List"=[0.0, 10.0], "Coefficients"=[2.656295322589486e-18, 0.9999999999999999], "Order"=1, "Algorithm"=enum."SVD", "Max Error % of Full Scale"=0.0, "Max Mean Squared Error"=0.0, "Use Error %"=FALSE, "Use MSE"=FALSE, "Allow Manual Entry"=FALSE, "Max Stability Error"=2.0, "Max Error % of Reading"=0.0, "Use Error % of Reading"=FALSE}, {"Sensor Name"="AI 7", "Sensor Info"={"Manufacturer"="", "Model"="", "Serial Number"=""}, "Last Cal Info"={"Last Calibration Date"=3154600502.2809997, "Calibrator"="", "Cal Duration"=0}, "Voltage Range"={"High Limit"=10.0, "Low Limit"=0.0}, "EGU Range"={"High Limit"=10.0, "Low Limit"=0.0}, "Units"="Volts", "Calibration Type"=enum."Calibrate Analog", "EGU List"=[0.0, 10.0], "Voltage List"=[0.0, 10.0], "Coefficients"=[2.656295322589486e-18, 0.9999999999999999], "Order"=1, "Algorithm"=enum."SVD", "Max Error % of Full Scale"=0.0, "Max Mean Squared Error"=0.0, "Use Error %"=FALSE, "Use MSE"=FALSE, "Allow Manual Entry"=FALSE, "Max Stability Error"=2.0, "Max Error % of Reading"=0.0, "Use Error % of Reading"=FALSE}, {"Sensor Name"="AI 8", "Sensor Info"={"Manufacturer"="", "Model"="", "Serial Number"=""}, "Last Cal Info"={"Last Calibration Date"=3154600511.7339997, "Calibrator"="", "Cal Duration"=0}, "Voltage Range"={"High Limit"=10.0, "Low Limit"=0.0}, "EGU Range"={"High Limit"=10.0, "Low Limit"=0.0}, "Units"="Volts", "Calibration Type"=enum."Calibrate Analog", "EGU List"=[0.0, 10.0], "Voltage List"=[0.0, 10.0], "Coefficients"=[2.656295322589486e-18, 0.9999999999999999], "Order"=1, "Algorithm"=enum."SVD", "Max Error % of Full Scale"=0.0, "Max Mean Squared Error"=0.0, "Use Error %"=FALSE, "Use MSE"=FALSE, "Allow Manual Entry"=FALSE, "Max Stability Error"=2.0, "Max Error % of Reading"=0.0, "Use Error % of Reading"=FALSE}, {"Sensor Name"="AI 9", "Sensor Info"={"Manufacturer"="", "Model"="", "Serial Number"=""}, "Last Cal Info"={"Last Calibration Date"=3154600521.89, "Calibrator"="", "Cal Duration"=0}, "Voltage Range"={"High Limit"=10.0, "Low Limit"=0.0}, "EGU Range"={"High Limit"=10.0, "Low Limit"=0.0}, "Units"="Volts", "Calibration Type"=enum."Calibrate Analog", "EGU List"=[0.0, 10.0], "Voltage List"=[0.0, 10.0], "Coefficients"=[-0.0, 1.0], "Order"=1, "Algorithm"=enum."SVD", "Max Error % of Full Scale"=0.0, "Max Mean Squared Error"=0.0, "Use Error %"=FALSE, "Use MSE"=FALSE, "Allow Manual Entry"=FALSE, "Max Stability Error"=2.0, "Max Error % of Reading"=0.0, "Use Error % of Reading"=FALSE}, {"Sensor Name"="Scott", "Sensor Info"={"Manufacturer"="", "Model"="", "Serial Number"=""}, "Last Cal Info"={"Last Calibration Date"=0.0, "Calibrator"="", "Cal Duration"=0}, "Voltage Range"={"High Limit"=10.0, "Low Limit"=-10.0}, "EGU Range"={"High Limit"=10.0, "Low Limit"=-10.0}, "Units"="Volts", "Calibration Type"=enum."Calibrate Analog", "EGU List"=[0.0, 10.0, 20.0], "Voltage List"=[0.0, 10.0, 20.0], "Coefficients"=[3.116871181724906e-15, 0.9999999999999998], "Order"=1, "Algorithm"=enum."SVD", "Max Error % of Full Scale"=0.0, "Max Mean Squared Error"=0.0, "Use Error %"=FALSE, "Use MSE"=FALSE, "Allow Manual Entry"=FALSE, "Max Stability Error"=2.0, "Max Error % of Reading"=0.0, "Use Error % of Reading"=FALSE}, {"Sensor Name"="Strain 0", "Sensor Info"={"Manufacturer"="", "Model"="", "Serial Number"=""}, "Last Cal Info"={"Last Calibration Date"=3154628048.187, "Calibrator"="", "Cal Duration"=0}, "Voltage Range"={"High Limit"=0.05, "Low Limit"=-0.05}, "EGU Range"={"High Limit"=10000.0, "Low Limit"=-10000.0}, "Units"="ue", "Calibration Type"=enum."Calibrate Analog", "EGU List"=[0.0, 139.98], "Voltage List"=[8.528640074655414e-05, -0.0014254050469025969], "Coefficients"=[7.9026000942022065, -92659.5567995229], "Order"=1, "Algorithm"=enum."SVD", "Max Error % of Full Scale"=0.0, "Max Mean Squared Error"=0.0, "Use Error %"=FALSE, "Use MSE"=FALSE, "Allow Manual Entry"=FALSE, "Max Stability Error"=2.0, "Max Error % of Reading"=0.0, "Use Error % of Reading"=FALSE}, {"Sensor Name"="Strain 1", "Sensor Info"={"Manufacturer"="", "Model"="", "Serial Number"=""}, "Last Cal Info"={"Last Calibration Date"=3154601435.546, "Calibrator"="", "Cal Duration"=0}, "Voltage Range"={"High Limit"=0.05, "Low Limit"=-0.05}, "EGU Range"={"High Limit"=10000.0, "Low Limit"=-10000.0}, "Units"="ue", "Calibration Type"=enum."Calibrate Analog", "EGU List"=[0.0, 198.39], "Voltage List"=[-0.001665323298657313, -0.0031823454801924527], "Coefficients"=[-217.784217819607, -130775.93881932605], "Order"=1, "Algorithm"=enum."SVD", "Max Error % of Full Scale"=0.0, "Max Mean Squared Error"=0.0, "Use Error %"=FALSE, "Use MSE"=FALSE, "Allow Manual Entry"=FALSE, "Max Stability Error"=2.0, "Max Error % of Reading"=0.0, "Use Error % of Reading"=FALSE}, {"Sensor Name"="Strain 10", "Sensor Info"={"Manufacturer"="", "Model"="", "Serial Number"=""}, "Last Cal Info"={"Last Calibration Date"=3155919669.421, "Calibrator"="", "Cal Duration"=0}, "Voltage Range"={"High Limit"=0.05, "Low Limit"=-0.05}, "EGU Range"={"High Limit"=10000.0, "Low Limit"=-10000.0}, "Units"="ue", "Calibration Type"=enum."Calibrate Analog", "EGU List"=[0.0, 198.39], "Voltage List"=[0.00928323432430625, 0.004247745492495596], "Coefficients"=[365.74420460721797, -39398.359648166115], "Order"=1, "Algorithm"=enum."SVD", "Max Error % of Full Scale"=0.0, "Max Mean Squared Error"=0.0, "Use Error %"=FALSE, "Use MSE"=FALSE, "Allow Manual Entry"=FALSE, "Max Stability Error"=2.0, "Max Error % of Reading"=0.0, "Use Error % of Reading"=FALSE}, {"Sensor Name"="Strain 11", "Sensor Info"={"Manufacturer"="", "Model"="", "Serial Number"=""}, "Last Cal Info"={"Last Calibration Date"=3155919688.9059997, "Calibrator"="", "Cal Duration"=0}, "Voltage Range"={"High Limit"=0.05, "Low Limit"=-0.05}, "EGU Range"={"High Limit"=10000.0, "Low Limit"=-10000.0}, "Units"="ue", "Calibration Type"=enum."Calibrate Analog", "EGU List"=[0.0, 198.39], "Voltage List"=[0.009270323118194937, 0.004226221022196114], "Coefficients"=[364.61185130998246, -39331.08335720854], "Order"=1, "Algorithm"=enum."SVD", "Max Error % of Full Scale"=0.0, "Max Mean Squared Error"=0.0, "Use Error %"=FALSE, "Use MSE"=FALSE, "Allow Manual Entry"=FALSE, "Max Stability Error"=2.0, "Max Error % of Reading"=0.0, "Use Error % of Reading"=FALSE}, {"Sensor Name"="Strain 12", "Sensor Info"={"Manufacturer"="", "Model"="", "Serial Number"=""}, "Last Cal Info"={"Last Calibration Date"=3155919703.5, "Calibrator"="", "Cal Duration"=0}, "Voltage Range"={"High Limit"=0.05, "Low Limit"=-0.05}, "EGU Range"={"High Limit"=10000.0, "Low Limit"=-10000.0}, "Units"="ue", "Calibration Type"=enum."Calibrate Analog", "EGU List"=[0.0, 10000.0], "Voltage List"=[0.009183059975504875, 0.00414156454987824], "Coefficients"=[18214.952509578965, -1983538.445590684], "Order"=1, "Algorithm"=enum."SVD", "Max Error % of Full Scale"=0.0, "Max Mean Squared Error"=0.0, "Use Error %"=FALSE, "Use MSE"=FALSE, "Allow Manual Entry"=FALSE, "Max Stability Error"=2.0, "Max Error % of Reading"=0.0, "Use Error % of Reading"=FALSE}, {"Sensor Name"="Strain 13", "Sensor Info"={"Manufacturer"="", "Model"="", "Serial Number"=""}, "Last Cal Info"={"Last Calibration Date"=3155919717.9839997, "Calibrator"="", "Cal Duration"=0}, "Voltage Range"={"High Limit"=0.05, "Low Limit"=-0.05}, "EGU Range"={"High Limit"=10000.0, "Low Limit"=-10000.0}, "Units"="ue", "Calibration Type"=enum."Calibrate Analog", "EGU List"=[0.0, 10000.0], "Voltage List"=[0.00907615415751934, 0.004033509385772049], "Coefficients"=[17998.797393722474, -1983086.3470747652], "Order"=1, "Algorithm"=enum."SVD", "Max Error % of Full Scale"=0.0, "Max Mean Squared Error"=0.0, "Use Error %"=FALSE, "Use MSE"=FALSE, "Allow Manual Entry"=FALSE, "Max Stability Error"=2.0, "Max Error % of Reading"=0.0, "Use Error % of Reading"=FALSE}, {"Sensor Name"="Strain 14", "Sensor Info"={"Manufacturer"="", "Model"="", "Serial Number"=""}, "Last Cal Info"={"Last Calibration Date"=3155919736.875, "Calibrator"="", "Cal Duration"=0}, "Voltage Range"={"High Limit"=0.05, "Low Limit"=-0.05}, "EGU Range"={"High Limit"=10000.0, "Low Limit"=-10000.0}, "Units"="ue", "Calibration Type"=enum."Calibrate Analog", "EGU List"=[0.0, 10000.0], "Voltage List"=[0.0092898035813123, 0.004254268301650882], "Coefficients"=[18448.49269318779, -1985886.1957317842], "Order"=1, "Algorithm"=enum."SVD", "Max Error % of Full Scale"=0.0, "Max Mean Squared Error"=0.0, "Use Error %"=FALSE, "Use MSE"=FALSE, "Allow Manual Entry"=FALSE, "Max Stability Error"=2.0, "Max Error % of Reading"=0.0, "Use Error % of Reading"=FALSE}, {"Sensor Name"="Strain 15", "Sensor Info"={"Manufacturer"="", "Model"="", "Serial Number"=""}, "Last Cal Info"={"Last Calibration Date"=3155919755.265, "Calibrator"="", "Cal Duration"=0}, "Voltage Range"={"High Limit"=0.05, "Low Limit"=-0.05}, "EGU Range"={"High Limit"=10000.0, "Low Limit"=-10000.0}, "Units"="ue", "Calibration Type"=enum."Calibrate Analog", "EGU List"=[0.0, 10000.0], "Voltage List"=[0.00911857127211988, 0.0040747079234570265], "Coefficients"=[18078.545435885466, -1982607.2414612575], "Order"=1, "Algorithm"=enum."SVD", "Max Error % of Full Scale"=0.0, "Max Mean Squared Error"=0.0, "Use Error %"=FALSE, "Use MSE"=FALSE, "Allow Manual Entry"=FALSE, "Max Stability Error"=2.0, "Max Error % of Reading"=0.0, "Use Error % of Reading"=FALSE}, {"Sensor Name"="Strain 2", "Sensor Info"={"Manufacturer"="", "Model"="", "Serial Number"=""}, "Last Cal Info"={"Last Calibration Date"=3154601463.2339997, "Calibrator"="", "Cal Duration"=0}, "Voltage Range"={"High Limit"=0.05, "Low Limit"=-0.05}, "EGU Range"={"High Limit"=10000.0, "Low Limit"=-10000.0}, "Units"="ue", "Calibration Type"=enum."Calibrate Analog", "EGU List"=[0.0, 198.39], "Voltage List"=[-0.01778510406240821, -0.019272710733115674], "Coefficients"=[-2371.8546470776187, -133361.86500538563], "Order"=1, "Algorithm"=enum."SVD", "Max Error % of Full Scale"=0.0, "Max Mean Squared Error"=0.0, "Use Error %"=FALSE, "Use MSE"=FALSE, "Allow Manual Entry"=FALSE, "Max Stability Error"=2.0, "Max Error % of Reading"=0.0, "Use Error % of Reading"=FALSE}, {"Sensor Name"="Strain 3", "Sensor Info"={"Manufacturer"="", "Model"="", "Serial Number"=""}, "Last Cal Info"={"Last Calibration Date"=3154601498.7809997, "Calibrator"="", "Cal Duration"=0}, "Voltage Range"={"High Limit"=0.05, "Low Limit"=-0.05}, "EGU Range"={"High Limit"=10000.0, "Low Limit"=-10000.0}, "Units"="ue", "Calibration Type"=enum."Calibrate Analog", "EGU List"=[0.0, 198.39], "Voltage List"=[-0.012857392450794577, -0.01438583350740373], "Coefficients"=[-1668.8756673234343, -129798.92102619135], "Order"=1, "Algorithm"=enum."SVD", "Max Error % of Full Scale"=0.0, "Max Mean Squared Error"=0.0, "Use Error %"=FALSE, "Use MSE"=FALSE, "Allow Manual Entry"=FALSE, "Max Stability Error"=2.0, "Max Error % of Reading"=0.0, "Use Error % of Reading"=FALSE}, {"Sensor Name"="Strain 4", "Sensor Info"={"Manufacturer"="", "Model"="", "Serial Number"=""}, "Last Cal Info"={"Last Calibration Date"=3155919563.265, "Calibrator"="", "Cal Duration"=0}, "Voltage Range"={"High Limit"=0.05, "Low Limit"=-0.05}, "EGU Range"={"High Limit"=10000.0, "Low Limit"=-10000.0}, "Units"="ue", "Calibration Type"=enum."Calibrate Analog", "EGU List"=[0.0, 198.39], "Voltage List"=[0.009254525888711214, 0.00421406074706465], "Coefficients"=[364.25316701260857, -39359.462752914136], "Order"=1, "Algorithm"=enum."SVD", "Max Error % of Full Scale"=0.0, "Max Mean Squared Error"=0.0, "Use Error %"=FALSE, "Use MSE"=FALSE, "Allow Manual Entry"=FALSE, "Max Stability Error"=2.0, "Max Error % of Reading"=0.0, "Use Error % of Reading"=FALSE}, {"Sensor Name"="Strain 5", "Sensor Info"={"Manufacturer"="", "Model"="", "Serial Number"=""}, "Last Cal Info"={"Last Calibration Date"=3155919582.453, "Calibrator"="", "Cal Duration"=0}, "Voltage Range"={"High Limit"=0.05, "Low Limit"=-0.05}, "EGU Range"={"High Limit"=10000.0, "Low Limit"=-10000.0}, "Units"="ue", "Calibration Type"=enum."Calibrate Analog", "EGU List"=[0.0, 198.39], "Voltage List"=[0.00942790717072785, 0.00438431843277067], "Coefficients"=[370.8475454242276, -39335.08664315769], "Order"=1, "Algorithm"=enum."SVD", "Max Error % of Full Scale"=0.0, "Max Mean Squared Error"=0.0, "Use Error %"=FALSE, "Use MSE"=FALSE, "Allow Manual Entry"=FALSE, "Max Stability Error"=2.0, "Max Error % of Reading"=0.0, "Use Error % of Reading"=FALSE}, {"Sensor Name"="Strain 6", "Sensor Info"={"Manufacturer"="", "Model"="", "Serial Number"=""}, "Last Cal Info"={"Last Calibration Date"=3155919598.7339997, "Calibrator"="", "Cal Duration"=0}, "Voltage Range"={"High Limit"=0.05, "Low Limit"=-0.05}, "EGU Range"={"High Limit"=10000.0, "Low Limit"=-10000.0}, "Units"="ue", "Calibration Type"=enum."Calibrate Analog", "EGU List"=[0.0, 198.39], "Voltage List"=[0.008921320913359523, 0.0038804980269633235], "Coefficients"=[351.11347807475505, -39356.66943097728], "Order"=1, "Algorithm"=enum."SVD", "Max Error % of Full Scale"=0.0, "Max Mean Squared Error"=0.0, "Use Error %"=FALSE, "Use MSE"=FALSE, "Allow Manual Entry"=FALSE, "Max Stability Error"=2.0, "Max Error % of Reading"=0.0, "Use Error % of Reading"=FALSE}, {"Sensor Name"="Strain 7", "Sensor Info"={"Manufacturer"="", "Model"="", "Serial Number"=""}, "Last Cal Info"={"Last Calibration Date"=3155919614.921, "Calibrator"="", "Cal Duration"=0}, "Voltage Range"={"High Limit"=0.05, "Low Limit"=-0.05}, "EGU Range"={"High Limit"=10000.0, "Low Limit"=-10000.0}, "Units"="ue", "Calibration Type"=enum."Calibrate Analog", "EGU List"=[0.0, 198.39], "Voltage List"=[0.009631765397265554, 0.004591415317729115], "Coefficients"=[379.1097655937529, -39360.36125852709], "Order"=1, "Algorithm"=enum."SVD", "Max Error % of Full Scale"=0.0, "Max Mean Squared Error"=0.0, "Use Error %"=FALSE, "Use MSE"=FALSE, "Allow Manual Entry"=FALSE, "Max Stability Error"=2.0, "Max Error % of Reading"=0.0, "Use Error % of Reading"=FALSE}, {"Sensor Name"="Strain 8", "Sensor Info"={"Manufacturer"="", "Model"="", "Serial Number"=""}, "Last Cal Info"={"Last Calibration Date"=3155919633.921, "Calibrator"="", "Cal Duration"=0}, "Voltage Range"={"High Limit"=0.05, "Low Limit"=-0.05}, "EGU Range"={"High Limit"=10000.0, "Low Limit"=-10000.0}, "Units"="ue", "Calibration Type"=enum."Calibrate Analog", "EGU List"=[0.0, 198.39], "Voltage List"=[0.009712127670645714, 0.004669082375243306], "Coefficients"=[382.06855098763407, -39339.32542324499], "Order"=1, "Algorithm"=enum."SVD", "Max Error % of Full Scale"=0.0, "Max Mean Squared Error"=0.0, "Use Error %"=FALSE, "Use MSE"=FALSE, "Allow Manual Entry"=FALSE, "Max Stability Error"=2.0, "Max Error % of Reading"=0.0, "Use Error % of Reading"=FALSE}, {"Sensor Name"="Strain 9", "Sensor Info"={"Manufacturer"="", "Model"="", "Serial Number"=""}, "Last Cal Info"={"Last Calibration Date"=3155919652.312, "Calibrator"="", "Cal Duration"=0}, "Voltage Range"={"High Limit"=0.05, "Low Limit"=-0.05}, "EGU Range"={"High Limit"=10000.0, "Low Limit"=-10000.0}, "Units"="ue", "Calibration Type"=enum."Calibrate Analog", "EGU List"=[0.0, 198.39], "Voltage List"=[0.009372463135048748, 0.0043335130205377935], "Coefficients"=[369.0060268720842, -39371.2966970411], "Order"=1, "Algorithm"=enum."SVD", "Max Error % of Full Scale"=0.0, "Max Mean Squared Error"=0.0, "Use Error %"=FALSE, "Use MSE"=FALSE, "Allow Manual Entry"=FALSE, "Max Stability Error"=2.0, "Max Error % of Reading"=0.0, "Use Error % of Reading"=FALSE}, {"Sensor Name"="WTI func gen", "Sensor Info"={"Manufacturer"="", "Model"="", "Serial Number"=""}, "Last Cal Info"={"Last Calibration Date"=3156162828.6089997, "Calibrator"="", "Cal Duration"=0}, "Voltage Range"={"High Limit"=10.0, "Low Limit"=-10.0}, "EGU Range"={"High Limit"=10.0, "Low Limit"=-10.0}, "Units"="Volts", "Calibration Type"=enum."Calibrate Analog", "EGU List"=[0.0, 10.0], "Voltage List"=[0.0, 10.0], "Coefficients"=[-0.0, 1.0], "Order"=1, "Algorithm"=enum."SVD", "Max Error % of Full Scale"=0.0, "Max Mean Squared Error"=0.0, "Use Error %"=FALSE, "Use MSE"=FALSE, "Allow Manual Entry"=FALSE, "Max Stability Error"=0.0, "Max Error % of Reading"=2.0, "Use Error % of Reading"=FALSE}, {"Sensor Name"="Chad Day", "Sensor Info"={"Manufacturer"="", "Model"="", "Serial Number"=""}, "Last Cal Info"={"Last Calibration Date"=0.0, "Calibrator"="", "Cal Duration"=0}, "Voltage Range"={"High Limit"=-0.05, "Low Limit"=0.05}, "EGU Range"={"High Limit"=0.0, "Low Limit"=135.0}, "Units"="", "Calibration Type"=enum."Calibrate Analog", "EGU List"=[0.0, 135.0], "Voltage List"=[-0.05, 0.05], "Coefficients"=[67.5, 1350.0], "Order"=1, "Algorithm"=enum."SVD", "Max Error % of Full Scale"=0.0, "Max Mean Squared Error"=0.0, "Use Error %"=FALSE, "Use MSE"=FALSE, "Allow Manual Entry"=FALSE, "Max Stability Error"=0.0, "Max Error % of Reading"=2.0, "Use Error % of Reading"=FALSE}], 13 "Channel index":i32) -> (4 "Sensor out":T4, 6 "OK Out":bool)   [LabVIEW 2023]
uses:
  Type Defs and Controls/Channel Config Screen.ctl
  Type Defs and Controls/Channel List.ctl
  Type Defs and Controls/System Type.ctl
  Type Defs and Controls/Ch Type.ctl
  <vilib>/Analysis/baseanly.llb/Mean (DBL).vi
  <vilib>/DAQmx/read.llb/DAQmx Read (Counter 1D DBL 1Chan NSamp).vi
  <vilib>/DAQmx/read.llb/DAQmx Read (Analog 2D DBL NChan NSamp).vi
  <vilib>/DAQmx/miscellaneous.llb/DAQmx Fill In Error Info.vi
  <vilib>/Analysis/NI_AALBase.lvlib
  <vilib>/Analysis/NI_AALPro.lvlib
  <resource>/objmgr/daqmx.rc
panel:
  out "Units":string
  in  "Voltage Range":cluster{"High Limit":dbl, "Low Limit":dbl} {"Low Limit" format="%_6f"; "High Limit" format="%_6f"}
  in  "Auto Shunt Cal":bool
  out "EGU":dbl format="%#8_5g"
  out "Volts":dbl format="%#8_5g"
  in  "Cancel":bool
  in  "OK":bool
  in  "Set Zero":bool
  in  "Zero":dbl
  out "Sensor":string
  out "Channel Name":string
  in  "Volts Tab":enum32{"Page 1", "Page 2"}(tab)
  in  "EGU High":dbl
  in  "Voltage Low":dbl
  in  "EGU Low":dbl
  in  "Acquire 1":bool
  in  "Acquire 2":bool
  in  "Span":dbl
  in  "Voltage High":dbl
  in  "Select Units":bool
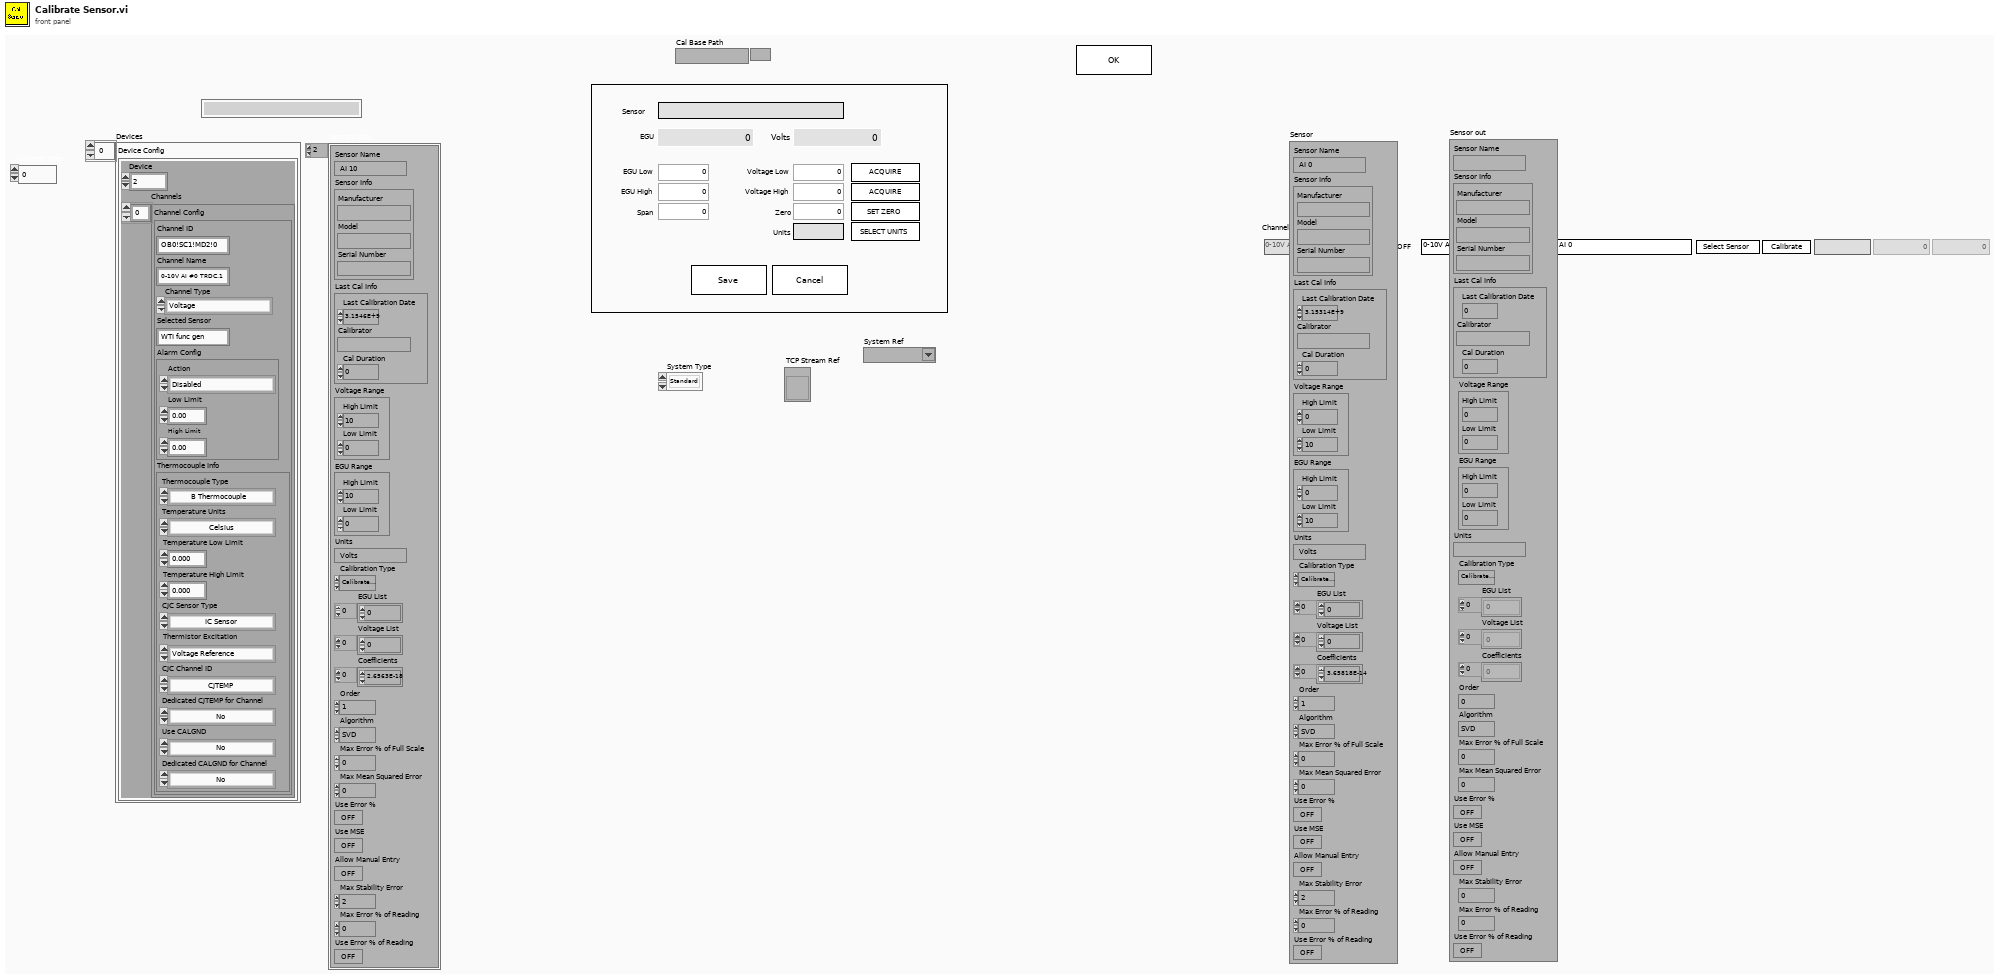
[diagram p1: front panel]
types:
  T1 = typedef "System Type.ctl" = enum16{"Standard", "Deformation", "Standard 8TC"}
  T2 = typedef "Channel List.ctl" = cluster{"Device":i16, "Channels":cluster{"Channel ID":string, "Channel Name":string, "Channel Type":enum16{"Voltage", "Thermocouple"}, "Selected Sensor":string, "Alarm Config":cluster{"Action":enum16{"Disabled", "Display On-Screen Warning", "Shutdown System"}, "Low Limit":dbl, "High Limit":dbl}, "Thermocouple Info":cluster{"Thermocouple Type":u16, "Temperature Units":u16, "Temperature Low Limit":sgl, "Temperature High Limit":sgl, "CJC Sensor Type":u16, "Thermistor Excitation":u16, "CJC Channel ID":u16, "Dedicated CJTEMP for Channel":u16, "Use CALGND":u16, "Dedicated CALGND for Channel":u16}}[]}[]
  T3 = cluster{"Sensor Name":string, "Sensor Info":cluster{"Manufacturer":string, "Model":string, "Serial Number":string}, "Last Cal Info":cluster{"Last Calibration Date":dbl, "Calibrator":string, "Cal Duration":i32}, "Voltage Range":cluster{"High Limit":dbl, "Low Limit":dbl}, "EGU Range":cluster{"High Limit":dbl, "Low Limit":dbl}, "Units":string, "Calibration Type":enum16{"Calibrate Analog", "Compare Analog Calibration"}, "EGU List":dbl[], "Voltage List":dbl[], "Coefficients":dbl[], "Order":i32, "Algorithm":enum32{"SVD", "Givens", "Givens2", "Householder", "LU Decomposition", "Cholesky"}, "Max Error % of Full Scale":dbl, "Max Mean Squared Error":dbl, "Use Error %":bool, "Use MSE":bool, "Allow Manual Entry":bool, "Max Stability Error":dbl, "Max Error % of Reading":dbl, "Use Error % of Reading":bool}[]
  T4 = cluster{"Sensor Name":string, "Sensor Info":cluster{"Manufacturer":string, "Model":string, "Serial Number":string}, "Last Cal Info":cluster{"Last Calibration Date":dbl, "Calibrator":string, "Cal Duration":i32}, "Voltage Range":cluster{"High Limit":dbl, "Low Limit":dbl}, "EGU Range":cluster{"High Limit":dbl, "Low Limit":dbl}, "Units":string, "Calibration Type":enum16{"Calibrate Analog", "Compare Analog Calibration"}, "EGU List":dbl[], "Voltage List":dbl[], "Coefficients":dbl[], "Order":i32, "Algorithm":enum32{"SVD", "Givens", "Givens2", "Householder", "LU Decomposition", "Cholesky"}, "Max Error % of Full Scale":dbl, "Max Mean Squared Error":dbl, "Use Error %":bool, "Use MSE":bool, "Allow Manual Entry":bool, "Max Stability Error":dbl, "Max Error % of Reading":dbl, "Use Error % of Reading":bool}
  T5 = typedef "Channel Config Screen.ctl" = cluster{"Channel":string, "Description":string, "Acquire":bool, "Sensor":string, "Chg Sensor":bool, "Cal Date":string, "Offset":dbl, "Span":dbl, "Cal":bool, "Test Limits":bool, "Type":string, "Data Index":u32}
  T6 = typedef "Ch Type.ctl" = enum16{"V", "A", "mA"}
  T7 = cluster{"Channel Info":T5, "Sensor":cluster{"Sensor Name":string, "Sensor Info":cluster{"Manufacturer":string, "Model":string, "Serial Number":string}, "Last Cal Info":cluster{"Last Calibration Date":dbl, "Calibrator":string, "Cal Duration":i32}, "Voltage Range":cluster{"High Limit":dbl, "Low Limit":dbl}, "EGU Range":cluster{"High Limit":dbl, "Low Limit":dbl}, "Units":string, "Calibration Type":enum16{"Calibrate Analog", "Compare Analog Calibration"}, "EGU List":dbl[], "Voltage List":dbl[], "Coefficients":dbl[], "Order":i32, "Algorithm":enum32{"SVD", "Givens", "Givens2", "Householder", "LU Decomposition", "Cholesky"}, "Max Error % of Full Scale":dbl, "Max Mean Squared Error":dbl, "Use Error %":bool, "Use MSE":bool, "Allow Manual Entry":bool, "Max Stability Error":dbl, "Max Error % of Reading":dbl, "Use Error % of Reading":bool}, "Devices":T2, "Sensors Info":cluster{"Sensor Name":string, "Sensor Info":cluster{"Manufacturer":string, "Model":string, "Serial Number":string}, "Last Cal Info":cluster{"Last Calibration Date":dbl, "Calibrator":string, "Cal Duration":i32}, "Voltage Range":cluster{"High Limit":dbl, "Low Limit":dbl}, "EGU Range":cluster{"High Limit":dbl, "Low Limit":dbl}, "Units":string, "Calibration Type":enum16{"Calibrate Analog", "Compare Analog Calibration"}, "EGU List":dbl[], "Voltage List":dbl[], "Coefficients":dbl[], "Order":i32, "Algorithm":enum32{"SVD", "Givens", "Givens2", "Householder", "LU Decomposition", "Cholesky"}, "Max Error % of Full Scale":dbl, "Max Mean Squared Error":dbl, "Use Error %":bool, "Use MSE":bool, "Allow Manual Entry":bool, "Max Stability Error":dbl, "Max Error % of Reading":dbl, "Use Error % of Reading":bool}[], "Channel index":i32, "DAQ Task":refnum<k21>, "Allow Shunt Cal":bool, "Coefficients":dbl[], "Cal sensor index":i32, "Channel ID":string, "Input limits":cluster{"High Limit":dbl, "Low Limit":dbl}, "Cal Base Path":path, "OK":bool, "AI Coeffs":cluster{"Coefficients":dbl[]}[], "Ch Type":T6, "TCP Stream Ref":refnum<vi>, "System Type":T1, "Ctr Present":bool, "Ctr Task":refnum<k21>, "System Ref":tag}
  T8 = enum8{"Enabled", "Disabled", "Disabled and Grayed Out"}
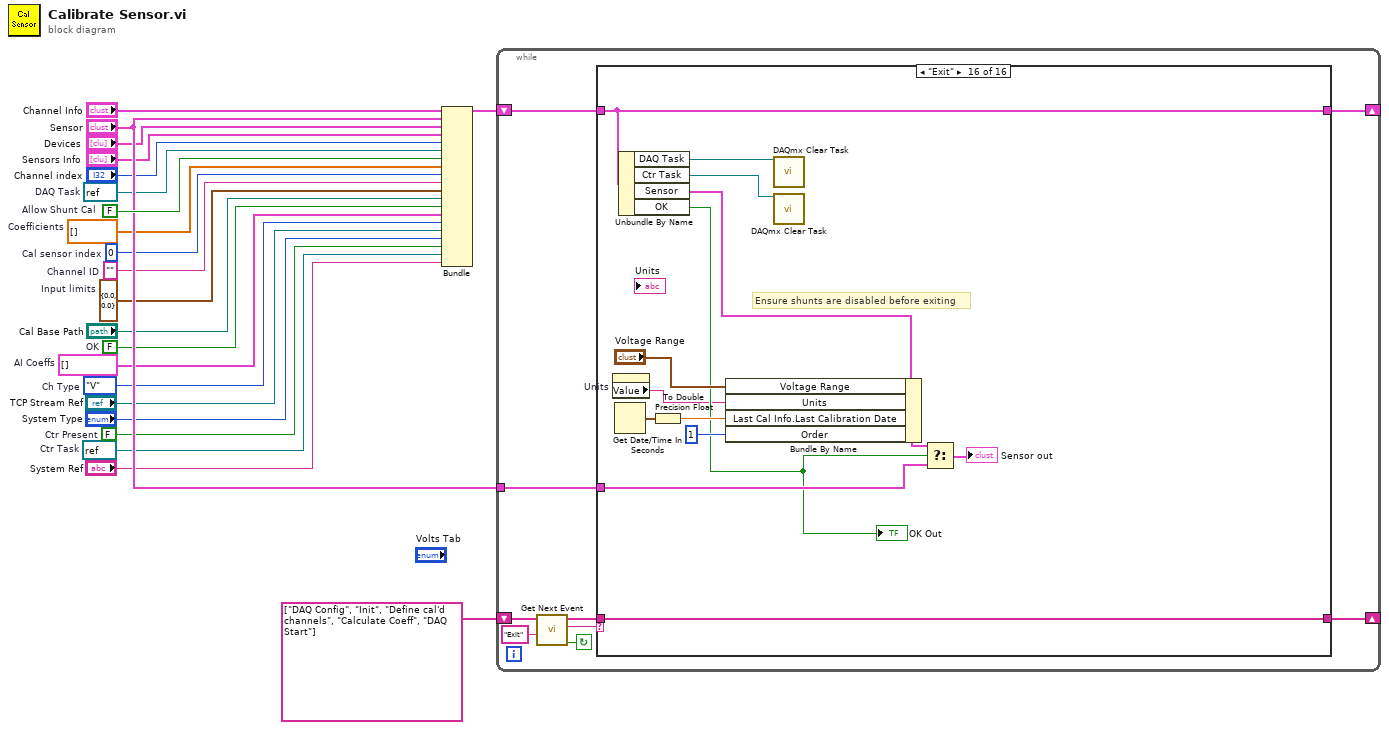
[diagram p0: block diagram]
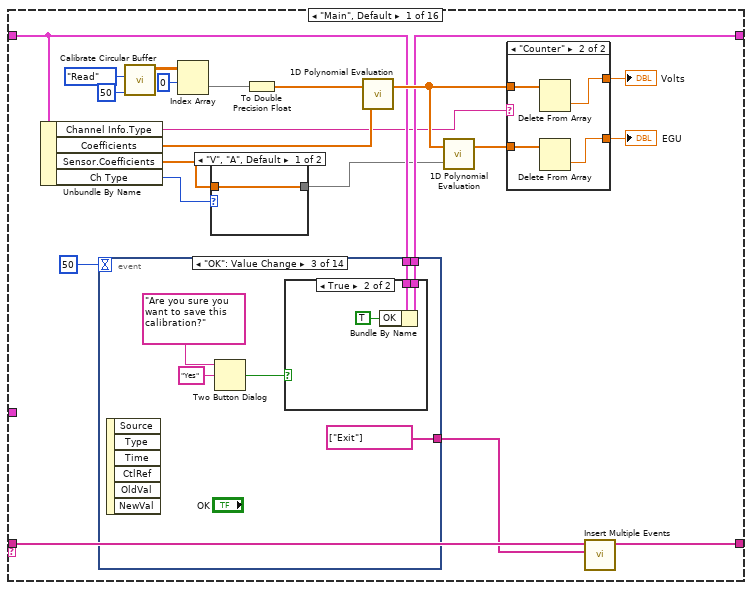
[diagram p2: hidden frame]
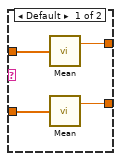
[diagram p3: hidden frame]
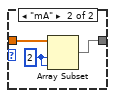
[diagram p4: hidden frame]
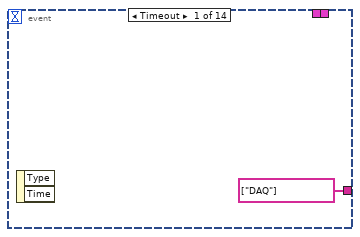
[diagram p5: hidden frame]
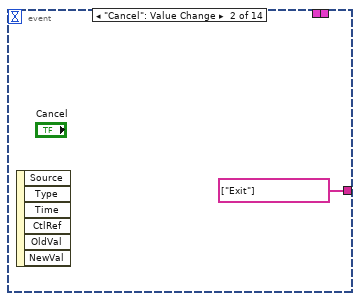
[diagram p6: hidden frame]
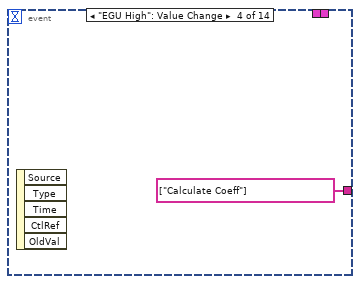
[diagram p8: hidden frame]
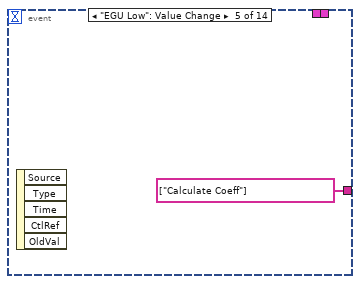
[diagram p9: hidden frame]
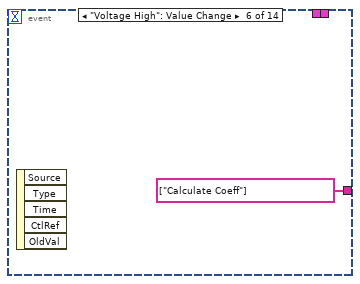
[diagram p10: hidden frame]
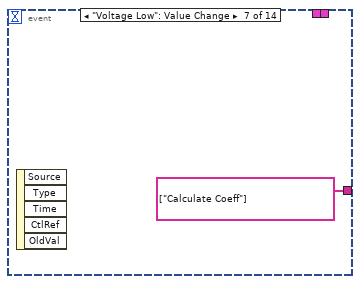
[diagram p11: hidden frame]
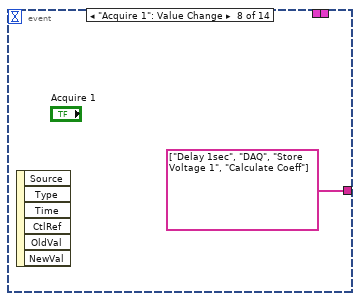
[diagram p12: hidden frame]
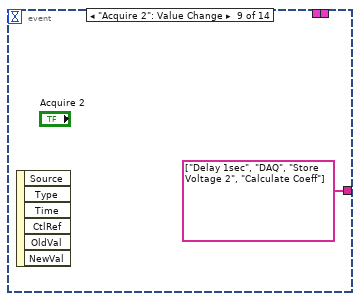
[diagram p13: hidden frame]
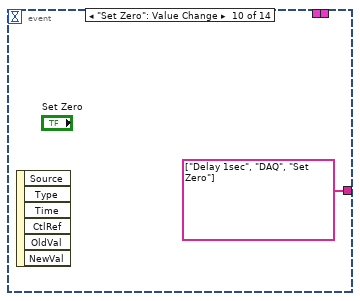
[diagram p14: hidden frame]
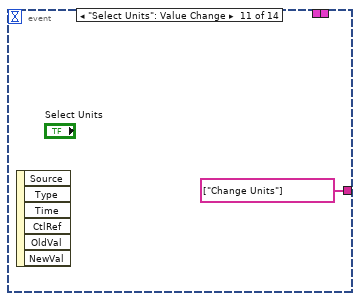
[diagram p15: hidden frame]
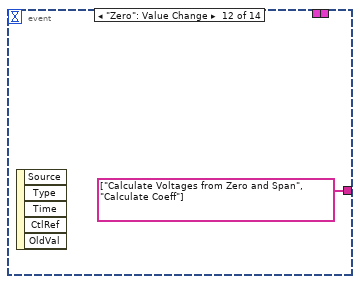
[diagram p16: hidden frame]
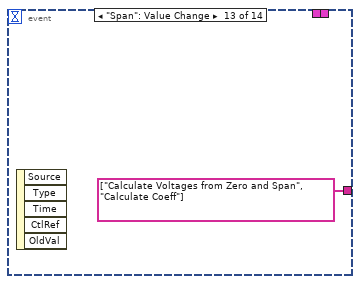
[diagram p17: hidden frame]
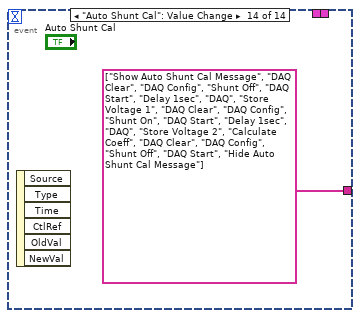
[diagram p18: hidden frame]
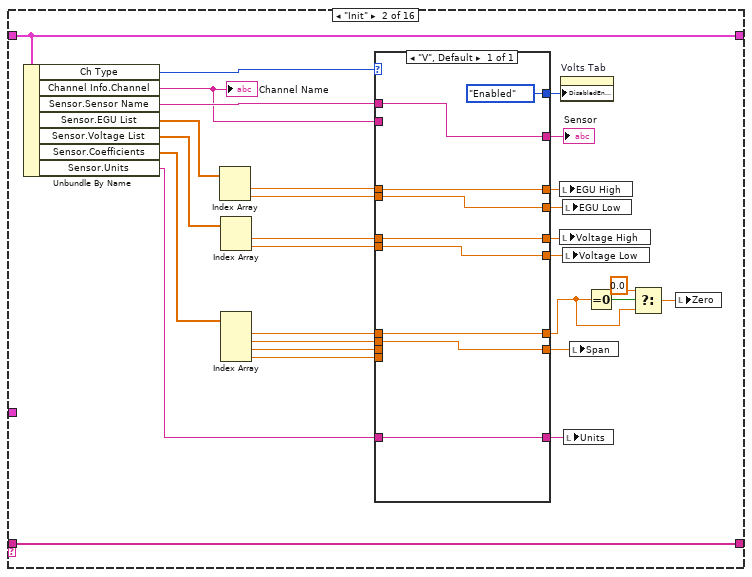
[diagram p19: hidden frame]
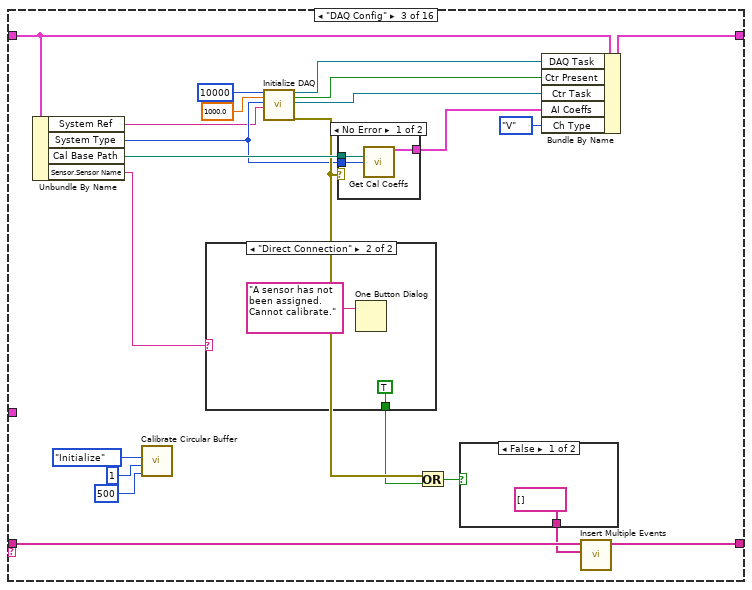
[diagram p20: hidden frame]
diagram:
  w2 = refnum<k21> refnum  # Ctr Task
  w3 = FALSE  # Ctr Present
  w6 = Ch_Type."V"  # Ch Type
  w7 = cluster{"Coefficients":dbl[]}[] []  # AI Coeffs
  w8 = FALSE  # OK
  w9 = refnum<k21> refnum  # DAQ Task
  w11 = dbl[] []  # Coefficients
  w12 = cluster{"High Limit":dbl, "Low Limit":dbl} {"High Limit"=0.0, "Low Limit"=0.0}  # Input limits
  w13 = ""  # Channel ID
  w17 = 0  # Cal sensor index
  w20 = FALSE  # Allow Shunt Cal
  n1 = Bundle("Channel Info"="Channel Info", "Sensor"="Sensor", "Devices"="Devices", "Sensors Info"="Sensors Info", "Channel index"="Channel index", "DAQ Task"=w9, "Allow Shunt Cal"=w20, "Coefficients"=w11, "Cal sensor index"=w17, "Channel ID"=w13, "Input limits"=w12, "Cal Base Path"="Cal Base Path", "OK"=w8, "AI Coeffs"=w7, "Ch Type"=w6, "TCP Stream Ref"="TCP Stream Ref", "System Type"="System Type", "Ctr Present"=w3, "Ctr Task"=w2, "System Ref"="System Ref") -> (w21:T7)  [unwired: 1 in]
  n2 = while {
    shift-left: string[] ["DAQ Config", "Init", "Define cal'd channels", "Calculate Coeff", "DAQ Start"] ("event queue out") -> [w29]
    shift-right: [w27] -> _
    shift-left: w21 -> [w28]
    shift-right: [w24] -> _
    tunnel: "Sensor" -> [w25]
    stop <- w31 continue-if-true
    n3 = call "Get Next Event.vi"("Exit Event"="Exit", "event queue in"=w29) -> ("Condition (Exit:F)"=w31:bool, "next event"=w30:string, "event queue out"=w23:string[])  [unwired: 3 in]
    n4 = case shown="\"Exit\"" w30 {
      tunnel: w28 -> [w38 w125 w153 w176 w181 w204 w207 w228 w230 w233 w237 w261 w270 w285 w289 w302]
      tunnel: [w52 w129 w149 w177 w185 w205 w209 w227 w231 w234 w244 w263 w272 w287 w288 w303] -> w27
      tunnel: w23 -> [w51 w129 w150 w177 w185 w205 w209 w227 w231 w234 w243 w263 w272 w287 w288 w303]
      tunnel: w25 -> [_ _ _ _ _ _ _ _ _ _ _ _ _ _ _ w301]
      tunnel: [w37 w125 w160 w175 w181 w204 w208 w228 w230 w233 w236 w262 w269 w286 w289 w302] -> w24
      frame "Main", Default {
        n5 = Unbundle By Name(w38) -> ("Channel Info.Type"=w32:string, "Coefficients"=w41:dbl[], "Sensor.Coefficients"=w34:dbl[], "Ch Type"=w35:T6)
        n6 = event shown="[2] \"OK\": Value Change" {
          selector: _ -> [_ _ _ _ _ _ _ _ _ _ _ _ _ _]
          dyn-events: _ -> [_ _ _ _ _ _ _ _ _ _ _ _ _ _]
          timeout: 50 -> [_ _ _ _ _ _ _ _ _ _ _ _ _ _]
          tunnel: [string[] ["DAQ"] ("Events to Insert") string[] ["Exit"] ("Events to Insert") string[] ["Exit"] ("Events to Insert") string[] ["Calculate Coeff"] ("Events to Insert") string[] ["Calculate Coeff"] ("Events to Insert") string[] ["Calculate Coeff"] ("Events to Insert") string[] ["Calculate Coeff"] ("Events to Insert") string[] ["Delay 1sec", "DAQ", "Store Voltage 1", "Calculate Coeff"] ("Events to Insert") string[] ["Delay 1sec", "DAQ", "Store Voltage 2", "Calculate Coeff"] ("Events to Insert") string[] ["Delay 1sec", "DAQ", "Set Zero"] ("Events to Insert") string[] ["Change Units"] ("Events to Insert") string[] ["Calculate Voltages from Zero and Span", "Calculate Coeff"] ("Events to Insert") string[] ["Calculate Voltages from Zero and Span", "Calculate Coeff"] ("Events to Insert") string[] ["Show Auto Shunt Cal Message", "DAQ Clear", "DAQ Config", "Shunt Off", "DAQ Start", "Delay 1sec", "DAQ", "Store Voltage 1", "DAQ Clear", "DAQ Config", "Shunt On", "DAQ Start", "Delay 1sec", "DAQ", "Store Voltage 2", "Calculate Coeff", "DAQ Clear", "DAQ Config", "Shunt Off", "DAQ Start", "Hide Auto Shunt Cal Message"] ("Events to Insert")] -> w50
          tunnel: w38 -> [w65 w67 w74 w79 w81 w83 w85 w87 w89 w91 w93 w95 w97 w99]
          tunnel: [w65 w67 w73 w79 w81 w83 w85 w87 w89 w91 w93 w95 w97 w99] -> w37
          event Timeout {
            n7 = event-data() -> ()  [unwired: 1 in, 2 out]
          }
          event "Cancel": Value Change {
            n8 = event-data() -> ()  [unwired: 1 in, 6 out]
          }
          event "OK": Value Change {
            n9 = event-data() -> ()  [unwired: 1 in, 6 out]
            n10 = Two Button Dialog(message="Are you sure you want to save this calibration?", 2:"Yes" ("T button name (\"OK\")")) -> (T button?=w70:bool)  [unwired: 1 in]
            n11 = case shown="True" w70 {
              tunnel: w74 -> [w75 w78]
              tunnel: [w75 w77] -> w73
              frame False {
              }
              frame True {
                n12 = Bundle By Name(cluster=w78, "OK"=TRUE) -> (w77:T7)
              }
            }
          }
          event "EGU High": Value Change {
            n13 = event-data() -> ()  [unwired: 1 in, 5 out]
          }
          event "EGU Low": Value Change {
            n14 = event-data() -> ()  [unwired: 1 in, 5 out]
          }
          event "Voltage High": Value Change {
            n15 = event-data() -> ()  [unwired: 1 in, 5 out]
          }
          event "Voltage Low": Value Change {
            n16 = event-data() -> ()  [unwired: 1 in, 5 out]
          }
          event "Acquire 1": Value Change {
            n17 = event-data() -> ()  [unwired: 1 in, 6 out]
          }
          event "Acquire 2": Value Change {
            n18 = event-data() -> ()  [unwired: 1 in, 6 out]
          }
          event "Set Zero": Value Change {
            n19 = event-data() -> ()  [unwired: 1 in, 6 out]
          }
          event "Select Units": Value Change {
            n20 = event-data() -> ()  [unwired: 1 in, 6 out]
          }
          event "Zero": Value Change {
            n21 = event-data() -> ()  [unwired: 1 in, 5 out]
          }
          event "Span": Value Change {
            n22 = event-data() -> ()  [unwired: 1 in, 5 out]
          }
          event "Auto Shunt Cal": Value Change {
            n23 = event-data() -> ()  [unwired: 1 in, 6 out]
          }
        }
        n24 = call "Calibrate Circular Buffer.vi"("# of Samples"=50, "Mode"=enum16{"Initialize", "Read", "Write"}."Read") -> ("Data Read"=w47:sgl[][])  [unwired: 7 in, 2 out]
        n25 = Index Array(array=w47, index (row)=0) -> (element=w40:sgl[])  [unwired: 1 in]
        n26 = case shown="\"V\", \"A\", Default" w35 {
          tunnel: [w61 w63] -> w33
          tunnel: w34 -> [w61 w64]
          frame "V", "A", Default {
          }
          frame "mA" {
            w62 = 2 ("index")
            n27 = Array Subset(array=w64, index=w62, length=w62) -> (w63:dbl[])
          }
        }
        n28 = To Double Precision Float(number=w40) -> (double precision float=w36:dbl[])
        n29 = call <vilib>:"1D Polynomial Evaluation.vi"("Coefficients: a"=w41, "X"=w36) -> ("Y"=w39:dbl[])  [unwired: 1 out]
        n30 = call <vilib>:"1D Polynomial Evaluation.vi"("Coefficients: a"=w33, "X"=w39) -> ("Y"=w43:dbl[])  [unwired: 1 out]
        n31 = case shown="\"Counter\"" w32 {
          tunnel: [w56 w59] -> w45
          tunnel: w43 -> [w55 w58]
          tunnel: [w54 w57] -> w42
          tunnel: w39 -> [w53 w60]
          frame Default {
            n32 = call-poly <vilib>:"Mean.vi"("X"=w53) -> ("mean"=w56:dbl)  [unwired: 1 out]
            n33 = call-poly <vilib>:"Mean.vi"("X"=w55) -> ("mean"=w54:dbl)  [unwired: 1 out]
          }
          frame "Counter" {
            n34 = Delete From Array(array=w60) -> (deleted portion=w59:dbl)  [unwired: 2 in, 1 out]
            n35 = Delete From Array(array=w58) -> (deleted portion=w57:dbl)  [unwired: 2 in, 1 out]
          }
        }
        "Volts" <- w45
        "EGU" <- w42
        n36 = call "Insert Multiple Events.vi"("Events to Insert"=w50, "Event queue in"=w51) -> ("Event queue out"=w52:string[])  [unwired: 5 in]
      }
      frame "Init" {
        n37 = Unbundle By Name(w125) -> ("Ch Type"=w124:T6, "Channel Info.Channel"=w114:string, "Sensor.Sensor Name"=w115:string, "Sensor.EGU List"=w128:dbl[], "Sensor.Voltage List"=w127:dbl[], "Sensor.Coefficients"=w126:dbl[], "Sensor.Units"=w122:string)
        "Channel Name" <- w114
        n38 = Index Array(array=w128) -> (element #1=w110:dbl, element #2=w107:dbl)  [unwired: 2 in]
        n39 = Index Array(array=w127) -> (element #1=w106:dbl, element #2=w103:dbl)  [unwired: 2 in]
        n40 = Index Array(array=w126) -> (element #1=w120:dbl, element #2=w119:dbl, element #3=w118:dbl, element #4=w117:dbl)  [unwired: 4 in]
        n41 = case shown="\"V\", Default" w124 {
          tunnel: [T8."Enabled" ("Disabled")] -> w123
          tunnel: [w137] -> w121
          tunnel: w122 -> [w137]
          tunnel: [w136] -> w111
          tunnel: w120 -> [w136]
          tunnel: [w135] -> w102
          tunnel: w119 -> [w135]
          tunnel: w118 -> [_]
          tunnel: w117 -> [_]
          tunnel: [w134] -> w116
          tunnel: w115 -> [w134]
          tunnel: w114 -> [_]
          tunnel: [w133] -> w109
          tunnel: w110 -> [w133]
          tunnel: [w132] -> w108
          tunnel: w107 -> [w132]
          tunnel: [w131] -> w105
          tunnel: w106 -> [w131]
          tunnel: [w130] -> w104
          tunnel: w103 -> [w130]
          frame "V", Default {
          }
        }
        "Sensor" <- w116
        n42 = local write "EGU High"(w109) -> ()
        n43 = local write "Voltage High"(w105) -> ()
        n44 = property on="Volts Tab" class="TabCtl (strict)"("DisabledEnum"=w123) -> ()  [unwired: 2 in, 2 out]
        n45 = local write "EGU Low"(w108) -> ()
        n46 = local write "Voltage Low"(w104) -> ()
        n47 = local write "Units"(w121) -> ()
        n48 = local write "Span"(w102) -> ()
        n49 = Equal To 0?(x=w111) -> (x = 0?=w112:bool)
        n50 = Select(t=0.0 ("Zero"), s=w112, f=w111) -> (s? t:f=w101:dbl)
        n51 = local write "Zero"(w101) -> ()
      }
      frame "DAQ Config" {
        n52 = Unbundle By Name(w153) -> ("System Ref"=w139:tag, "System Type"=w144:T1, "Cal Base Path"=w152:path, "Sensor.Sensor Name"=w145:string)
        n53 = call "Calibrate Circular Buffer.vi"("# of Samples"=500, "# of Channels"=1, "Mode"=enum16{"Initialize", "Read", "Write"}."Initialize") -> ()  [unwired: 6 in, 3 out]
        n54 = case shown="\"Direct Connection\"" w145 {
          tunnel: [FALSE TRUE] -> w146
          frame Default {
          }
          frame "Direct Connection" {
            n55 = One Button Dialog(message="A sensor has not been assigned.  Cannot calibrate.") -> ()  [unwired: 1 in, 1 out]
          }
        }
        n56 = call "Initialize DAQ.vi"("number of samples"=10000, "rate"=1000.0, "System Type"=w144, "System Ref"=w139) -> ("AI Task OUT"=w154:refnum<k21>, "Ctr Present"=w141:bool, "Ctr Task OUT"=w140:refnum<k21>, "error out"=w147:errorcluster)  [unwired: 12 in]
        n57 = case shown="No Error" w147 {
          tunnel: w152 -> [w168 _]
          tunnel: [w167 cluster{"Coefficients":dbl[]}[] [] ("AI Coeffs")] -> w151
          tunnel: w144 -> [w166 _]
          frame No Error {
            n58 = call "Get Cal Coeffs.vi"("Cal Files Path"=w168, "System Type"=w166) -> ("AI Coeffs"=w167:cluster{"Coefficients":dbl[]}[])  [unwired: 12 in, 1 out]
          }
          frame Error {
          }
        }
        n59 = Or(x=w147, y=w146) -> (x .or. y?=w142:bool)
        n60 = case shown="False" w142 {
          tunnel: [string[] [] ("Events to Insert") string[] ["Exit"] ("Events to Insert")] -> w143
          frame False {
          }
          frame True {
          }
        }
        n61 = Bundle By Name(cluster=w153, "DAQ Task"=w154, "Ctr Present"=w141, "Ctr Task"=w140, "AI Coeffs"=w151, "Ch Type"=Ch_Type."V") -> (w160:T7)
        n62 = call "Insert Multiple Events.vi"("Events to Insert"=w143, "Event queue in"=w150) -> ("Event queue out"=w149:string[])  [unwired: 5 in]
      }
      frame "DAQ Start" {
        n63 = Unbundle By Name(w176) -> ("DAQ Task"=w171:refnum<k21>)
        n64 = call "Calibrate Circular Buffer.vi"("# of Samples"=100, "# of Channels"=1, "Mode"=enum16{"Initialize", "Read", "Write"}."Initialize") -> ()  [unwired: 6 in, 3 out]
        n65 = call <vilib>:"DAQmx Start Task.vi"("task/channels in"=w171) -> ("task out"=w170:refnum<k21>)  [unwired: 13 in, 1 out]
        n66 = Bundle By Name(cluster=w176, "DAQ Task"=w170) -> (w175:T7)
      }
      frame "DAQ" {
        n67 = Unbundle By Name(w181) -> ("DAQ Task"=w184:refnum<k21>, "Ctr Task"=w179:refnum<k21>, "Ctr Present"=w178:bool, "Channel Info.Data Index"=w180:u32)
        n68 = property class="DAQmx Read"(reference=w184) -> (reference out=w182:refnum<k21>, "AvailSampPerChan"=w183:u32)  [unwired: 1 in, 1 out]
        n69 = case shown="1, Default" w183 {
          selector: w183 -> [_ w190]
          tunnel: w182 -> [_ w195]
          tunnel: w180 -> [_ w194]
          tunnel: w179 -> [_ w191]
          tunnel: w178 -> [_ w186]
          frame 0 {
          }
          frame 1, Default {
            n70 = case shown="True" w186 {
              tunnel: w191 -> [_ w201]
              tunnel: w190 -> [_ w200]
              tunnel: [dbl[] [] ("data") w199] -> w188
              frame False {
              }
              frame True {
                n71 = call-poly <vilib>:"DAQmx Read.vi"("task/channels in"=w201, "number of samples per channel"=w200) -> ("data"=w199:dbl[])  [unwired: 11 in, 2 out]
              }
            }
            n72 = call-poly <vilib>:"DAQmx Read.vi"("task/channels in"=w195, "number of samples per channel"=w190) -> ("data"=w189:dbl[][])  [unwired: 11 in, 2 out]
            n73 = Build Array (concatenate)(w189, w188) -> (w187:dbl[][])
            n74 = Array Subset(array=w187, index (row)=w194, length (row)=1 ("length")) -> (w192:dbl[][])  [unwired: 2 in]
            n75 = Transpose 2D Array(2D array=w192) -> (transposed array=w196:dbl[][])
            n76 = call "Calibrate Circular Buffer.vi"("Mode"=enum16{"Initialize", "Read", "Write"}."Write", "Data to Write"=w196) -> ()  [unwired: 7 in, 3 out]
          }
        }
      }
      frame "DAQ Clear" {
        n77 = Unbundle By Name(w204) -> ("DAQ Task"=w203:refnum<k21>, "Ctr Task"=w202:refnum<k21>)
        n78 = call <vilib>:"DAQmx Clear Task.vi"("task in"=w203) -> ()  [unwired: 14 in, 1 out]
        n79 = call <vilib>:"DAQmx Clear Task.vi"("task in"=w202) -> ()  [unwired: 14 in, 1 out]
      }
      frame "Calculate Coeff" {
        n80 = Unbundle By Name(w207) -> ("Ch Type"=w206:T6)
        n81 = case shown="\"V\"" w206 {
          tunnel: [w210 w225] -> w208
          tunnel: w207 -> [w210 w221]
          frame Default {
          }
          frame "V" {
            # "^ Removes negative sign before 0"
            n82 = Build Array("EGU High", "EGU Low") -> (w224:dbl[])
            n83 = Build Array("Voltage High", "Voltage Low") -> (w223:dbl[])
            n84 = call <vilib>:"Linear Fit Coefficients.vi"("Y"=w224, "X"=w223) -> ("slope"=w212:dbl, "intercept"=w211:dbl)  [unwired: 11 in, 1 out]
            n85 = Equal To 0?(x=w211) -> (x = 0?=w215:bool)
            n86 = Select(t=0.0 ("Zero"), s=w215, f=w211) -> (s? t:f=w213:dbl)
            n87 = Build Array(w213, w212) -> (w220:dbl[])
            n88 = local write "Span"(w212) -> ()
            n89 = local write "Zero"(w211) -> ()
            n90 = Bundle By Name(cluster=w221, "Sensor.EGU List"=w224, "Sensor.Voltage List"=w223, "Sensor.Coefficients"=w220, "Sensor.Order"=1) -> (w225:T7)
          }
        }
      }
      frame "Delay 1sec" {
        n91 = Wait (ms)(milliseconds to wait=u32 1000) -> ()  [unwired: 1 out]
      }
      frame "Store Voltage 1" {
        n92 = local read "Volts"() -> (w229:dbl)
        n93 = local write "Voltage High"(w229) -> ()
      }
      frame "Store Voltage 2" {
        n94 = local read "Volts"() -> (w232:dbl)
        n95 = local write "Voltage Low"(w232) -> ()
      }
      frame "Set Zero" {
        n96 = Unbundle By Name(w237) -> ("Sensor.Coefficients"=w238:dbl[], "Ch Type"=w240:T6)
        n97 = local read "Volts"() -> (w239:dbl)
        n98 = case shown="\"V\", Default" w240 {
          tunnel: [w246 w247 w252] -> w241
          tunnel: w239 -> [w246 w248 w253]
          tunnel: w238 -> [w245 w250 w255]
          tunnel: [w245 w249 w254] -> w235
          frame "V", Default {
          }
          frame "A" {
            n99 = Negate(x=w248) -> (-x=w247:dbl)
            n100 = Replace Array Subset(array=w250, new element=w247, index=0) -> (w249:dbl[])
          }
          frame "mA" {
            n101 = Negate(x=w253) -> (-x=w252:dbl)
            n102 = Replace Array Subset(array=w255, new element=w252, index=2) -> (w254:dbl[])
          }
        }
        n103 = local write "Zero"(w241) -> ()
        n104 = Bundle By Name(cluster=w237, "Sensor.Coefficients"=w235) -> (w236:T7)
        n105 = call "Insert Multiple Events.vi"("Events to Insert"=string[] ["Calculate Voltages from Zero and Span", "Calculate Coeff"], "Event queue in"=w243) -> ("Event queue out"=w244:string[])  [unwired: 5 in]
      }
      frame "Change Units" {
        n106 = Unbundle By Name(w261) -> ("Sensor.Units"=w260:string)
        n107 = call "Select Units.vi"() -> ("Element"=w258:string, "Cancelled"=w259:bool)  [unwired: 4 in]
        n108 = Select(t=w260, s=w259, f=w258) -> (s? t:f=w257:string)
        n109 = local write "Units"(w257) -> ()
        n110 = Bundle By Name(cluster=w261, "Sensor.Units"=w257) -> (w262:T7)
      }
      frame "Calculate Voltages from Zero and Span" {
        n111 = Unbundle By Name(w270) -> ("Sensor.EGU List"=w271:dbl[])
        n112 = for {
          tunnel: w271 -> [w277] mode=indexing
          tunnel: [w275] -> w268 mode=indexing
          tunnel: "Zero" -> [w276]
          tunnel: "Span" -> [w273]
          n113 = Subtract(x=w277, y=w276) -> (x-y=w274:dbl)
          n114 = Divide(x=w274, y=w273) -> (x/y=w275:dbl)
        }
        n115 = Index Array(array=w268) -> (element #1=w267:dbl, element #2=w266:dbl)  [unwired: 2 in]
        n116 = local write "Voltage High"(w267) -> ()
        n117 = local write "Voltage Low"(w266) -> ()
        n118 = Bundle By Name(cluster=w270, "Sensor.Voltage List"=w268) -> (w269:T7)
      }
      frame "Define cal'd channels" {
        n119 = Unbundle By Name(w285) -> ("Channel Info.Channel"=w281:string, "AI Coeffs"=w279:cluster{"Coefficients":dbl[]}[])
        n120 = Match Pattern(string=w281, regular expression="-") -> (after substring=w283:string)  [unwired: 1 in, 3 out]
        n121 = Decimal String To Number(string=w283) -> (number=w278:i32)  [unwired: 2 in, 1 out]
        n122 = Index Array(array=w279, index=w278) -> (element=w282:cluster{"Coefficients":dbl[]})
        n123 = Unbundle(w282) -> ("Coefficients"=w280:dbl[])
        n124 = Bundle By Name(cluster=w285, "Channel ID"=w281, "Coefficients"=w280) -> (w286:T7)
      }
      frame "Blank" {
        # "Blank case template"
      }
      frame "Exit" {
        # "Ensure shunts are disabled before exiting"
        n125 = property on="Units" class="Str"() -> ("Value"=w291:string)  [unwired: 2 in, 2 out]
        n126 = Get Date/Time In Seconds() -> (seconds since 1Jan1904=w297:timestamp)
        n127 = Unbundle By Name(w302) -> ("DAQ Task"=w293:refnum<k21>, "Ctr Task"=w290:refnum<k21>, "Sensor"=w299:T4, "OK"=w292:bool)
        "OK Out" <- w292
        n128 = To Double Precision Float(number=w297) -> (double precision float=w296:dbl)
        n129 = Bundle By Name(cluster=w299, "Voltage Range"="Voltage Range", "Units"=w291, "Last Cal Info.Last Calibration Date"=w296, "Order"=1) -> (w298:T4)
        n130 = call <vilib>:"DAQmx Clear Task.vi"("task in"=w293) -> ()  [unwired: 14 in, 1 out]
        n131 = call <vilib>:"DAQmx Clear Task.vi"("task in"=w290) -> ()  [unwired: 14 in, 1 out]
        n132 = Select(t=w298, s=w292, f=w301) -> (s? t:f=→"Sensor out":T4)
      }
    }
  }
